vi "30XX.VI"() -> ()   [LabVIEW 2015]
uses:
  board.vis/Globals.vi
  <vilib>/Analysis/NI_AALBase.lvlib
panel:
  in  "send all":bool
  in  "Offset ADC 8":u16=49000
  in  "Offset ADC 3":u16=49000
  in  "Offset ADC 7":u16=49000
  in  "Offset ADC 2":u16=49000
  in  "Offset ADC 6":u16=49000
  in  "Offset ADC 1":u16=49000
  in  "Offset ADC 5":u16=49000
  in  "Offset ADC 4":u16=49000
  in  "custom pattern: 14bits (hex)":fxp<+,14,14>=100.0 format="%x"
  out "data adr  0x25":u16 format="%x"
  out "data adr  0x26":u16 format="%x"
  out "custom pattern: 14bits (dec)":fxp<+,14,14>
  in  "ADC mode":enum32{"1", "2", "3"}(radio)=enum."3"
  out "Signalverlaufgraph Cam 2":u16[](graph)=[28, 28, 29, 29, 30, 30, 31, 31, 32, 32, 33, 33, 34, 34, 35, 35, 36, 36, 37, 37, 38, 38, 39, 39, 40, 40, 41, 41, 42, 42, 43, 43, 44, 44, 45, 45, 46, 46, 47, 47, 48, 48, 49, 49, 50, 50, 51, 51, 52, 52, 53, 53, 54, 54, 55, 55, 56, 56, 57, 57, 58, 58, 59, 59, 60, 60, 61, 61, 62, 62, 63, 63, 64, 64, 65, 65, 66, 66, 67, 67, 68, 68, 69, 69, 70, 70, 71, 71, 72, 72, 73, 73, 74, 74, 75, 75, 76, 76, 77, 77, 78, 78, 79, 79, 80, 80, 81, 81, 82, 82, 83, 83, 84, 84, 85, 85, 86, 86, 87, 87, 88, 88, 89, 89, 90, 90, 91, 91, 92, 92, 93, 93, 94, 94, 95, 95, 96, 96, 97, 97, 98, 98, 99, 99, 100, 100, 101, 101, 102, 102, 103, 103, 104, 104, 105, 105, 106, 106, 107, 107, 108, 108, 109, 109, 110, 110, 111, 111, 112, 112, 113, 113, 114, 114, 115, 115, 116, 116, 117, 117, 118, 118, 119, 119, 120, 120, 121, 121, 122, 122, 123, 123, 124, 124, 125, 125, 126, 126, 127, 127, 128, 128, 129, 129, 130, 130, 131, 131, 132, 132, 133, 133, 134, 134, 135, 135, 136, 136, 137, 137, 138, 138, 139, 139, 140, 140, 141, 141, 142, 142, 143, 143, 144, 144, 145, 145, 146, 146, 147, 147, 148, 148, 149, 149, 150, 150, 151, 151, 152, 152, 153, 153, 154, 154, 155, 155, 156, 156, 157, 157, 158, 158, 159, 159, 160, 160, 161, 161, 162, 162, 163, 163, 164, 164, 165, 165, 166, 166, 167, 167, 168, 168, 169, 169, 170, 170, 171, 171, 172, 172, 173, 173, 174, 174, 175, 175, 176, 176, 177, 177, 178, 178, 179, 179, 180, 180, 181, 181, 182, 182, 183, 183, 184, 184, 185, 185, 186, 186, 187, 187, 188, 188, 189, 189, 190, 190, 191, 191, 192, 192, 193, 193, 194, 194, 195, 195, 196, 196, 197, 197, 198, 198, 199, 199, 200, 200, 201, 201, 202, 202, 203, 203, 204, 204, 205, 205, 206, 206, 207, 207, 208, 208, 209, 209, 210, 210, 211, 211, 212, 212, 213, 213, 214, 214, 215, 215, 216, 216, 217, 217, 218, 218, 219, 219, 220, 220, 221, 221, 222, 222, 223, 223, 224, 224, 225, 225, 226, 226, 227, 227, 228, 228, 229, 229, 230, 230, 231, 231, 232, 232, 233, 233, 234, 234, 235, 235, 236, 236, 237, 237, 238, 238, 239, 239, 240, 240, 241, 241, 242, 242, 243, 243, 244, 244, 245, 245, 246, 246, 247, 247, 248, 248, 249, 249, 250, 250, 251, 251, 252, 252, 253, 253, 254, 254, 255, 255, 256, 256, 257, 257, 258, 258, 259, 259, 260, 260, 261, 261, 262, 262, 263, 263, 264, 264, 265, 265, 266, 266, 267, 267, 268, 268, 269, 269, 270, 270, 271, 271, 272, 272, 273, 273, 274, 274, 275, 275, 276, 276, 277, 277, 278, 278, 279, 279, 280, 280, 281, 281, 282, 282, 283, 283, 284, 284, 285, 285, 286, 286, 287, 287, 288, 288, 289, 289, 290, 290, 291, 291, 292, 292, 293, 293, 294, 294, 295, 295, 296, 296, 297, 297, 298, 298, 299, 299, 300, 300, 301, 301, 302, 302, 303, 303, 304, 304, 305, 305, 306, 306, 307, 307, 308, 308, 309, 309, 310, 310, 311, 311, 312, 312, 313, 313, 314, 314, 315, 315, 316, 316, 317, 317, 318, 318, 319, 319, 320, 320, 321, 321, 322, 322, 323, 323, 324, 324, 325, 325, 326, 326, 327, 327, 328, 328, 329, 329, 330, 330, 331, 331, 332, 332, 333, 333, 334, 334, 335, 335, 336, 336, 337, 337, 338, 338, 339, 339, 340, 340, 341, 341, 342, 342, 343, 343, 344, 344, 345, 345, 346, 346, 347, 347, 348, 348, 349, 349, 350, 350, 351, 351, 352, 352, 353, 353, 354, 354, 355, 355, 356, 356, 357, 357, 358, 358, 359, 359, 360, 360, 361, 361, 362, 362, 363, 363, 364, 364, 365, 365, 366, 366, 367, 367, 368, 368, 369, 369, 370, 370, 371, 371, 372, 372, 373, 373, 374, 374, 375, 375, 376, 376, 377, 377, 378, 378, 379, 379, 380, 380, 381, 381, 382, 382, 383, 383, 384, 384, 385, 385, 386, 386, 387, 387, 388, 388, 389, 389, 390, 390, 391, 391, 392, 392, 393, 393, 394, 394, 395, 395, 396, 396, 397, 397, 398, 398, 399, 399, 400, 400, 401, 401, 402, 402, 403, 403, 404, 404, 405, 405, 406, 406, 407, 407, 408, 408, 409, 409, 410, 410, 411, 411, 412, 412, 413, 413, 414, 414, 415, 415, 416, 416, 417, 417, 418, 418, 419, 419, 420, 420, 421, 421, 422, 422, 423, 423, 424, 424, 425, 425, 426, 426, 427, 427, 428, 428, 429, 429, 430, 430, 431, 431, 432, 432, 433, 433, 434, 434, 435, 435, 436, 436, 437, 437, 438, 438, 439, 439, 440, 440, 441, 441, 442, 442, 443, 443, 444, 444, 445, 445, 446, 446, 447, 447, 448, 448, 449, 449, 450, 450, 451, 451, 452, 452, 453, 453, 454, 454, 455, 455, 456, 456, 457, 457, 458, 458, 459, 459, 460, 460, 461, 461, 462, 462, 463, 463, 464, 464, 465, 465, 466, 466, 467, 467, 468, 468, 469, 469, 470, 470, 471, 471, 472, 472, 473, 473, 474, 474, 475, 475, 476, 476, 477, 477, 478, 478, 479, 479, 480, 480, 481, 481, 482, 482, 483, 483, 484, 484, 485, 485, 486, 486, 487, 487, 488, 488, 489, 489, 490, 490, 491, 491, 492, 492, 493, 493, 494, 494, 495, 495, 496, 496, 497, 497, 498, 498, 499, 499, 500, 500, 501, 501, 502, 502, 503, 503, 504, 504, 505, 505, 506, 506, 507, 507, 508, 508, 509, 509, 510, 510, 511, 511, 512, 512, 513, 513, 514, 514, 515, 515, 516, 516, 517, 517, 518, 518, 519, 519, 520, 520, 521, 521, 522, 522, 523, 523, 524, 524, 525, 525, 526, 526, 527, 527, 528, 528, 529, 529, 530, 530, 531, 531, 532, 532, 533, 533, 534, 534, 535, 535, 536, 536, 537, 537, 538, 538, 539, 539, 540, 540, 541, 541, 542, 542, 543, 543, 544, 544, 544, 544, 544, 544, 544, 544, 544, 544, 544, 544, 544, 544, 544, 544, 544, 544, 544, 544, 544, 544, 544, 544, 544, 544, 544, 544, 544, 544, 544, 544, 544, 544, 544, 544, 544, 544, 544, 544, 544, 544, 544, 544, 544, 544, 544, 544, 544, 544, 544, 544, 544, 544, 544, 544]
  in  "extTrig":bool
  in  "ext. trig. slope":enum32{"1", "2", "3"}(radio)
  out "tRMS":dbl format="%0#.1f"
  out "mean":dbl=100.0 format="%#_4f"
  in  "rms_pixel":u16=100
  in  "is FFT":bool=TRUE
  in  "IR gain":bool
  in  "continuous":bool
  out "curr.block":u8=2
  out "Measure ON":bool
  in  "Board select\n1: board 1\n2: board 2\n3: both boards":u8=3
  in  "no.of blocks (nob)\npress enter":u32=4
  in  "block":u32(slide)=2 max=10 scale=0.9..4.0
  out "Signalverlaufgraph Board 2":u16[](graph)=[0, 0, 543, 543, 0, 1, 0, 0, 2, 2, 3, 3, 4, 4, 5, 5, 6, 6, 7, 7, 8, 8, 9, 9, 10, 10, 11, 11, 12, 12, 13, 13, 14, 14, 15, 15, 16, 16, 17, 17, 18, 18, 19, 19, 20, 20, 21, 21, 22, 22, 23, 23, 24, 24, 25, 25, 26, 26, 27, 27, 28, 28, 29, 29, 30, 30, 31, 31, 32, 32, 33, 33, 34, 34, 35, 35, 36, 36, 37, 37, 38, 38, 39, 39, 40, 40, 41, 41, 42, 42, 43, 43, 44, 44, 45, 45, 46, 46, 47, 47, 48, 48, 49, 49, 50, 50, 51, 51, 52, 52, 53, 53, 54, 54, 55, 55, 56, 56, 57, 57, 58, 58, 59, 59, 60, 60, 61, 61, 62, 62, 63, 63, 64, 64, 65, 65, 66, 66, 67, 67, 68, 68, 69, 69, 70, 70, 71, 71, 72, 72, 73, 73, 74, 74, 75, 75, 76, 76, 77, 77, 78, 78, 79, 79, 80, 80, 81, 81, 82, 82, 83, 83, 84, 84, 85, 85, 86, 86, 87, 87, 88, 88, 89, 89, 90, 90, 91, 91, 92, 92, 93, 93, 94, 94, 95, 95, 96, 96, 97, 97, 98, 98, 99, 99, 100, 100, 101, 101, 102, 102, 103, 103, 104, 104, 105, 105, 106, 106, 107, 107, 108, 108, 109, 109, 110, 110, 111, 111, 112, 112, 113, 113, 114, 114, 115, 115, 116, 116, 117, 117, 118, 118, 119, 119, 120, 120, 121, 121, 122, 122, 123, 123, 124, 124, 125, 125, 126, 126, 127, 127, 128, 128, 129, 129, 130, 130, 131, 131, 132, 132, 133, 133, 134, 134, 135, 135, 136, 136, 137, 137, 138, 138, 139, 139, 140, 140, 141, 141, 142, 142, 143, 143, 144, 144, 145, 145, 146, 146, 147, 147, 148, 148, 149, 149, 150, 150, 151, 151, 152, 152, 153, 153, 154, 154, 155, 155, 156, 156, 157, 157, 158, 158, 159, 159, 160, 160, 161, 161, 162, 162, 163, 163, 164, 164, 165, 165, 166, 166, 167, 167, 168, 168, 169, 169, 170, 170, 171, 171, 172, 172, 173, 173, 174, 174, 175, 175, 176, 176, 177, 177, 178, 178, 179, 179, 180, 180, 181, 181, 182, 182, 183, 183, 184, 184, 185, 185, 186, 186, 187, 187, 188, 188, 189, 189, 190, 190, 191, 191, 192, 192, 193, 193, 194, 194, 195, 195, 196, 196, 197, 197, 198, 198, 199, 199, 200, 200, 201, 201, 202, 202, 203, 203, 204, 204, 205, 205, 206, 206, 207, 207, 208, 208, 209, 209, 210, 210, 211, 211, 212, 212, 213, 213, 214, 214, 215, 215, 216, 216, 217, 217, 218, 218, 219, 219, 220, 220, 221, 221, 222, 222, 223, 223, 224, 224, 225, 225, 226, 226, 227, 227, 228, 228, 229, 229, 230, 230, 231, 231, 232, 232, 233, 233, 234, 234, 235, 235, 236, 236, 237, 237, 238, 238, 239, 239, 240, 240, 241, 241, 242, 242, 243, 243, 244, 244, 245, 245, 246, 246, 247, 247, 248, 248, 249, 249, 250, 250, 251, 251, 252, 252, 253, 253, 254, 254, 255, 255, 256, 256, 257, 257, 258, 258, 259, 259, 260, 260, 261, 261, 262, 262, 263, 263, 264, 264, 265, 265, 266, 266, 267, 267, 268, 268, 269, 269, 270, 270, 271, 271, 272, 272, 273, 273, 274, 274, 275, 275, 276, 276, 277, 277, 278, 278, 279, 279, 280, 280, 281, 281, 282, 282, 283, 283, 284, 284, 285, 285, 286, 286, 287, 287, 288, 288, 289, 289, 290, 290, 291, 291, 292, 292, 293, 293, 294, 294, 295, 295, 296, 296, 297, 297, 298, 298, 299, 299, 300, 300, 301, 301, 302, 302, 303, 303, 304, 304, 305, 305, 306, 306, 307, 307, 308, 308, 309, 309, 310, 310, 311, 311, 312, 312, 313, 313, 314, 314, 315, 315, 316, 316, 317, 317, 318, 318, 319, 319, 320, 320, 321, 321, 322, 322, 323, 323, 324, 324, 325, 325, 326, 326, 327, 327, 328, 328, 329, 329, 330, 330, 331, 331, 332, 332, 333, 333, 334, 334, 335, 335, 336, 336, 337, 337, 338, 338, 339, 339, 340, 340, 341, 341, 342, 342, 343, 343, 344, 344, 345, 345, 346, 346, 347, 347, 348, 348, 349, 349, 350, 350, 351, 351, 352, 352, 353, 353, 354, 354, 355, 355, 356, 356, 357, 357, 358, 358, 359, 359, 360, 360, 361, 361, 362, 362, 363, 363, 364, 364, 365, 365, 366, 366, 367, 367, 368, 368, 369, 369, 370, 370, 371, 371, 372, 372, 373, 373, 374, 374, 375, 375, 376, 376, 377, 377, 378, 378, 379, 379, 380, 380, 381, 381, 382, 382, 383, 383, 384, 384, 385, 385, 386, 386, 387, 387, 388, 388, 389, 389, 390, 390, 391, 391, 392, 392, 393, 393, 394, 394, 395, 395, 396, 396, 397, 397, 398, 398, 399, 399, 400, 400, 401, 401, 402, 402, 403, 403, 404, 404, 405, 405, 406, 406, 407, 407, 408, 408, 409, 409, 410, 410, 411, 411, 412, 412, 413, 413, 414, 414, 415, 415, 416, 416, 417, 417, 418, 418, 419, 419, 420, 420, 421, 421, 422, 422, 423, 423, 424, 424, 425, 425, 426, 426, 427, 427, 428, 428, 429, 429, 430, 430, 431, 431, 432, 432, 433, 433, 434, 434, 435, 435, 436, 436, 437, 437, 438, 438, 439, 439, 440, 440, 441, 441, 442, 442, 443, 443, 444, 444, 445, 445, 446, 446, 447, 447, 448, 448, 449, 449, 450, 450, 451, 451, 452, 452, 453, 453, 454, 454, 455, 455, 456, 456, 457, 457, 458, 458, 459, 459, 460, 460, 461, 461, 462, 462, 463, 463, 464, 464, 465, 465, 466, 466, 467, 467, 468, 468, 469, 469, 470, 470, 471, 471, 472, 472, 473, 473, 474, 474, 475, 475, 476, 476, 477, 477, 478, 478, 479, 479, 480, 480, 481, 481, 482, 482, 483, 483, 484, 484, 485, 485, 486, 486, 487, 487, 488, 488, 489, 489, 490, 490, 491, 491, 492, 492, 493, 493, 494, 494, 495, 495, 496, 496, 497, 497, 498, 498, 499, 499, 500, 500, 501, 501, 502, 502, 503, 503, 504, 504, 505, 505, 506, 506, 507, 507, 508, 508, 509, 509, 510, 510, 511, 511, 512, 512, 513, 513, 514, 514, 515, 515, 516, 516, 517, 517, 518, 518, 519, 519, 520, 520, 521, 521, 522, 522, 523, 523, 524, 524, 525, 525, 526, 526, 527, 527, 528, 528, 529, 529, 530, 530, 531, 531, 532, 532, 533, 533, 534, 534, 535, 535, 536, 536, 537, 537, 538, 538, 539, 539, 540, 540, 541, 541]
  out "Signalverlaufgraph":u16[](graph)=[544, 544, 545, 545, 49152, 2, 0, 762, 2, 2, 3, 3, 4, 4, 5, 5, 6, 6, 7, 7, 8, 8, 9, 9, 10, 10, 11, 11, 12, 12, 13, 13, 14, 14, 15, 15, 16, 16, 17, 17, 18, 18, 19, 19, 20, 20, 21, 21, 22, 22, 23, 23, 24, 24, 25, 25, 26, 26, 27, 27, 28, 28, 29, 29, 30, 30, 31, 31, 32, 32, 33, 33, 34, 34, 35, 35, 36, 36, 37, 37, 38, 38, 39, 39, 40, 40, 41, 41, 42, 42, 43, 43, 44, 44, 45, 45, 46, 46, 47, 47, 48, 48, 49, 49, 50, 50, 51, 51, 52, 52, 53, 53, 54, 54, 55, 55, 56, 56, 57, 57, 58, 58, 59, 59, 60, 60, 61, 61, 62, 62, 63, 63, 64, 64, 65, 65, 66, 66, 67, 67, 68, 68, 69, 69, 70, 70, 71, 71, 72, 72, 73, 73, 74, 74, 75, 75, 76, 76, 77, 77, 78, 78, 79, 79, 80, 80, 81, 81, 82, 82, 83, 83, 84, 84, 85, 85, 86, 86, 87, 87, 88, 88, 89, 89, 90, 90, 91, 91, 92, 92, 93, 93, 94, 94, 95, 95, 96, 96, 97, 97, 98, 98, 99, 99, 100, 100, 101, 101, 102, 102, 103, 103, 104, 104, 105, 105, 106, 106, 107, 107, 108, 108, 109, 109, 110, 110, 111, 111, 112, 112, 113, 113, 114, 114, 115, 115, 116, 116, 117, 117, 118, 118, 119, 119, 120, 120, 121, 121, 122, 122, 123, 123, 124, 124, 125, 125, 126, 126, 127, 127, 128, 128, 129, 129, 130, 130, 131, 131, 132, 132, 133, 133, 134, 134, 135, 135, 136, 136, 137, 137, 138, 138, 139, 139, 140, 140, 141, 141, 142, 142, 143, 143, 144, 144, 145, 145, 146, 146, 147, 147, 148, 148, 149, 149, 150, 150, 151, 151, 152, 152, 153, 153, 154, 154, 155, 155, 156, 156, 157, 157, 158, 158, 159, 159, 160, 160, 161, 161, 162, 162, 163, 163, 164, 164, 165, 165, 166, 166, 167, 167, 168, 168, 169, 169, 170, 170, 171, 171, 172, 172, 173, 173, 174, 174, 175, 175, 176, 176, 177, 177, 178, 178, 179, 179, 180, 180, 181, 181, 182, 182, 183, 183, 184, 184, 185, 185, 186, 186, 187, 187, 188, 188, 189, 189, 190, 190, 191, 191, 192, 192, 193, 193, 194, 194, 195, 195, 196, 196, 197, 197, 198, 198, 199, 199, 200, 200, 201, 201, 202, 202, 203, 203, 204, 204, 205, 205, 206, 206, 207, 207, 208, 208, 209, 209, 210, 210, 211, 211, 212, 212, 213, 213, 214, 214, 215, 215, 216, 216, 217, 217, 218, 218, 219, 219, 220, 220, 221, 221, 222, 222, 223, 223, 224, 224, 225, 225, 226, 226, 227, 227, 228, 228, 229, 229, 230, 230, 231, 231, 232, 232, 233, 233, 234, 234, 235, 235, 236, 236, 237, 237, 238, 238, 239, 239, 240, 240, 241, 241, 242, 242, 243, 243, 244, 244, 245, 245, 246, 246, 247, 247, 248, 248, 249, 249, 250, 250, 251, 251, 252, 252, 253, 253, 254, 254, 255, 255, 256, 256, 257, 257, 258, 258, 259, 259, 260, 260, 261, 261, 262, 262, 263, 263, 264, 264, 265, 265, 266, 266, 267, 267, 268, 268, 269, 269, 270, 270, 271, 271, 272, 272, 273, 273, 274, 274, 275, 275, 276, 276, 277, 277, 278, 278, 279, 279, 280, 280, 281, 281, 282, 282, 283, 283, 284, 284, 285, 285, 286, 286, 287, 287, 288, 288, 289, 289, 290, 290, 291, 291, 292, 292, 293, 293, 294, 294, 295, 295, 296, 296, 297, 297, 298, 298, 299, 299, 300, 300, 301, 301, 302, 302, 303, 303, 304, 304, 305, 305, 306, 306, 307, 307, 308, 308, 309, 309, 310, 310, 311, 311, 312, 312, 313, 313, 314, 314, 315, 315, 316, 316, 317, 317, 318, 318, 319, 319, 320, 320, 321, 321, 322, 322, 323, 323, 324, 324, 325, 325, 326, 326, 327, 327, 328, 328, 329, 329, 330, 330, 331, 331, 332, 332, 333, 333, 334, 334, 335, 335, 336, 336, 337, 337, 338, 338, 339, 339, 340, 340, 341, 341, 342, 342, 343, 343, 344, 344, 345, 345, 346, 346, 347, 347, 348, 348, 349, 349, 350, 350, 351, 351, 352, 352, 353, 353, 354, 354, 355, 355, 356, 356, 357, 357, 358, 358, 359, 359, 360, 360, 361, 361, 362, 362, 363, 363, 364, 364, 365, 365, 366, 366, 367, 367, 368, 368, 369, 369, 370, 370, 371, 371, 372, 372, 373, 373, 374, 374, 375, 375, 376, 376, 377, 377, 378, 378, 379, 379, 380, 380, 381, 381, 382, 382, 383, 383, 384, 384, 385, 385, 386, 386, 387, 387, 388, 388, 389, 389, 390, 390, 391, 391, 392, 392, 393, 393, 394, 394, 395, 395, 396, 396, 397, 397, 398, 398, 399, 399, 400, 400, 401, 401, 402, 402, 403, 403, 404, 404, 405, 405, 406, 406, 407, 407, 408, 408, 409, 409, 410, 410, 411, 411, 412, 412, 413, 413, 414, 414, 415, 415, 416, 416, 417, 417, 418, 418, 419, 419, 420, 420, 421, 421, 422, 422, 423, 423, 424, 424, 425, 425, 426, 426, 427, 427, 428, 428, 429, 429, 430, 430, 431, 431, 432, 432, 433, 433, 434, 434, 435, 435, 436, 436, 437, 437, 438, 438, 439, 439, 440, 440, 441, 441, 442, 442, 443, 443, 444, 444, 445, 445, 446, 446, 447, 447, 448, 448, 449, 449, 450, 450, 451, 451, 452, 452, 453, 453, 454, 454, 455, 455, 456, 456, 457, 457, 458, 458, 459, 459, 460, 460, 461, 461, 462, 462, 463, 463, 464, 464, 465, 465, 466, 466, 467, 467, 468, 468, 469, 469, 470, 470, 471, 471, 472, 472, 473, 473, 474, 474, 475, 475, 476, 476, 477, 477, 478, 478, 479, 479, 480, 480, 481, 481, 482, 482, 483, 483, 484, 484, 485, 485, 486, 486, 487, 487, 488, 488, 489, 489, 490, 490, 491, 491, 492, 492, 493, 493, 494, 494, 495, 495, 496, 496, 497, 497, 498, 498, 499, 499, 500, 500, 501, 501, 502, 502, 503, 503, 504, 504, 505, 505, 506, 506, 507, 507, 508, 508, 509, 509, 510, 510, 511, 511, 512, 512, 513, 513, 514, 514, 515, 515, 516, 516, 517, 517, 518, 518, 519, 519, 520, 520, 521, 521, 522, 522, 523, 523, 524, 524, 525, 525, 526, 526, 527, 527, 528, 528, 529, 529, 530, 530, 531, 531, 532, 532, 533, 533, 534, 534, 535, 535, 536, 536, 537, 537, 538, 538, 539, 539, 540, 540, 541, 541]
  out "boards recognised":u8=1
  in  "alloc mem":bool
  out "FREE \nRAM MB":dbl=15821.3046875
  out "BUILT-IN\nRAM MB":dbl=18096.171875
  out "SEC":dbl=0.44
  out "MB RAM":dbl=18.26171875
  in  "DAT in 10ns":u32
  in  "stop all":bool
  in  "start":bool
  in  "sample":u32(slide)=382 max=3000 scale=0.9..1100.0
  in  "no.of samples (nos)":u32=1100
  in  "exposuretime[ms]":dbl=0.1 format="%.3f"
  # "press Esc to stop measurement"
  # "exit here"
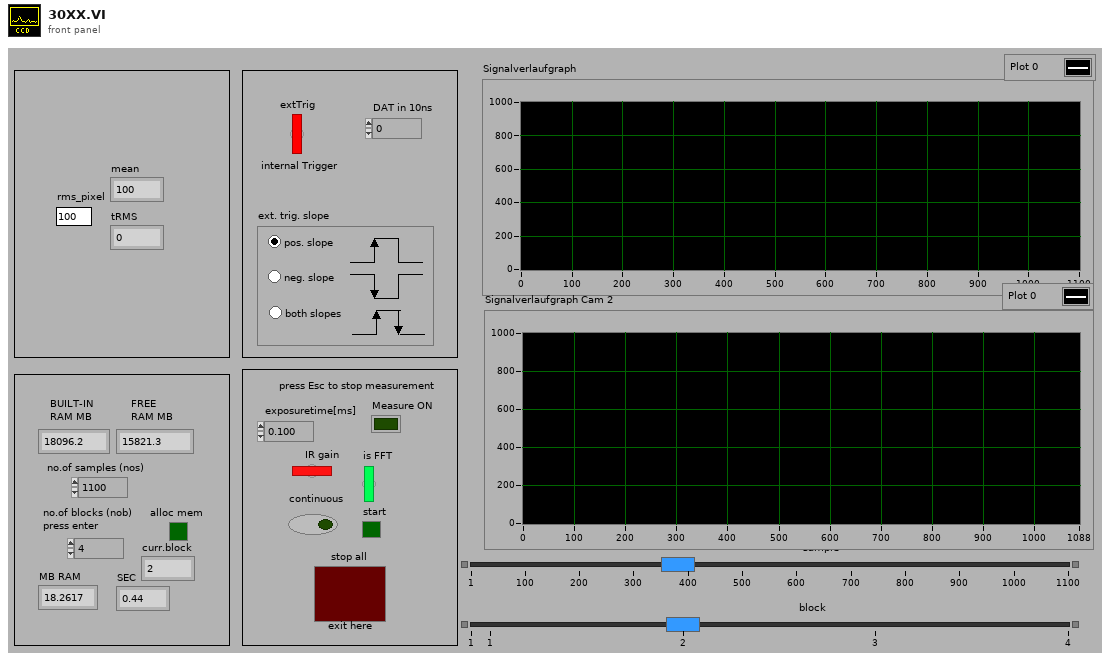
[diagram p1: front panel]
types:
  T1 = enum8{"Enabled", "Disabled", "Disabled and Grayed Out"}
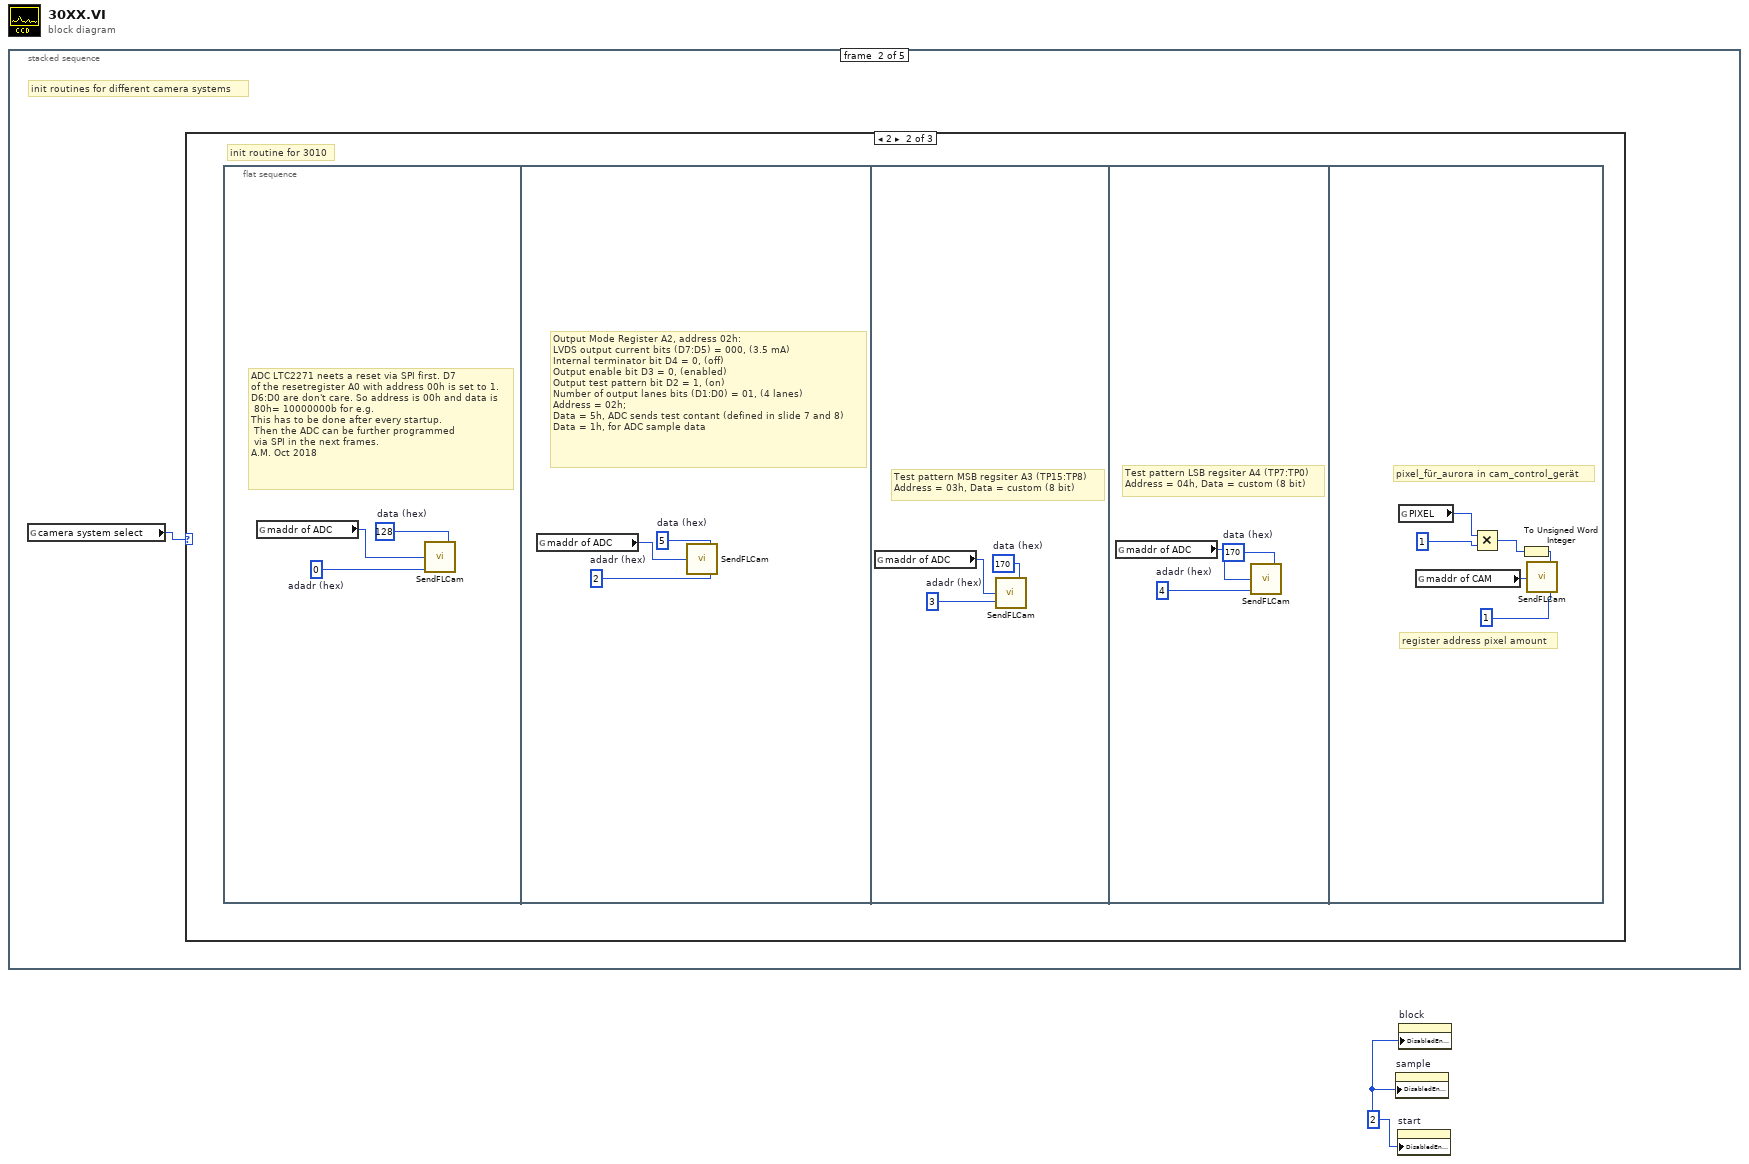
[diagram p0: block diagram]
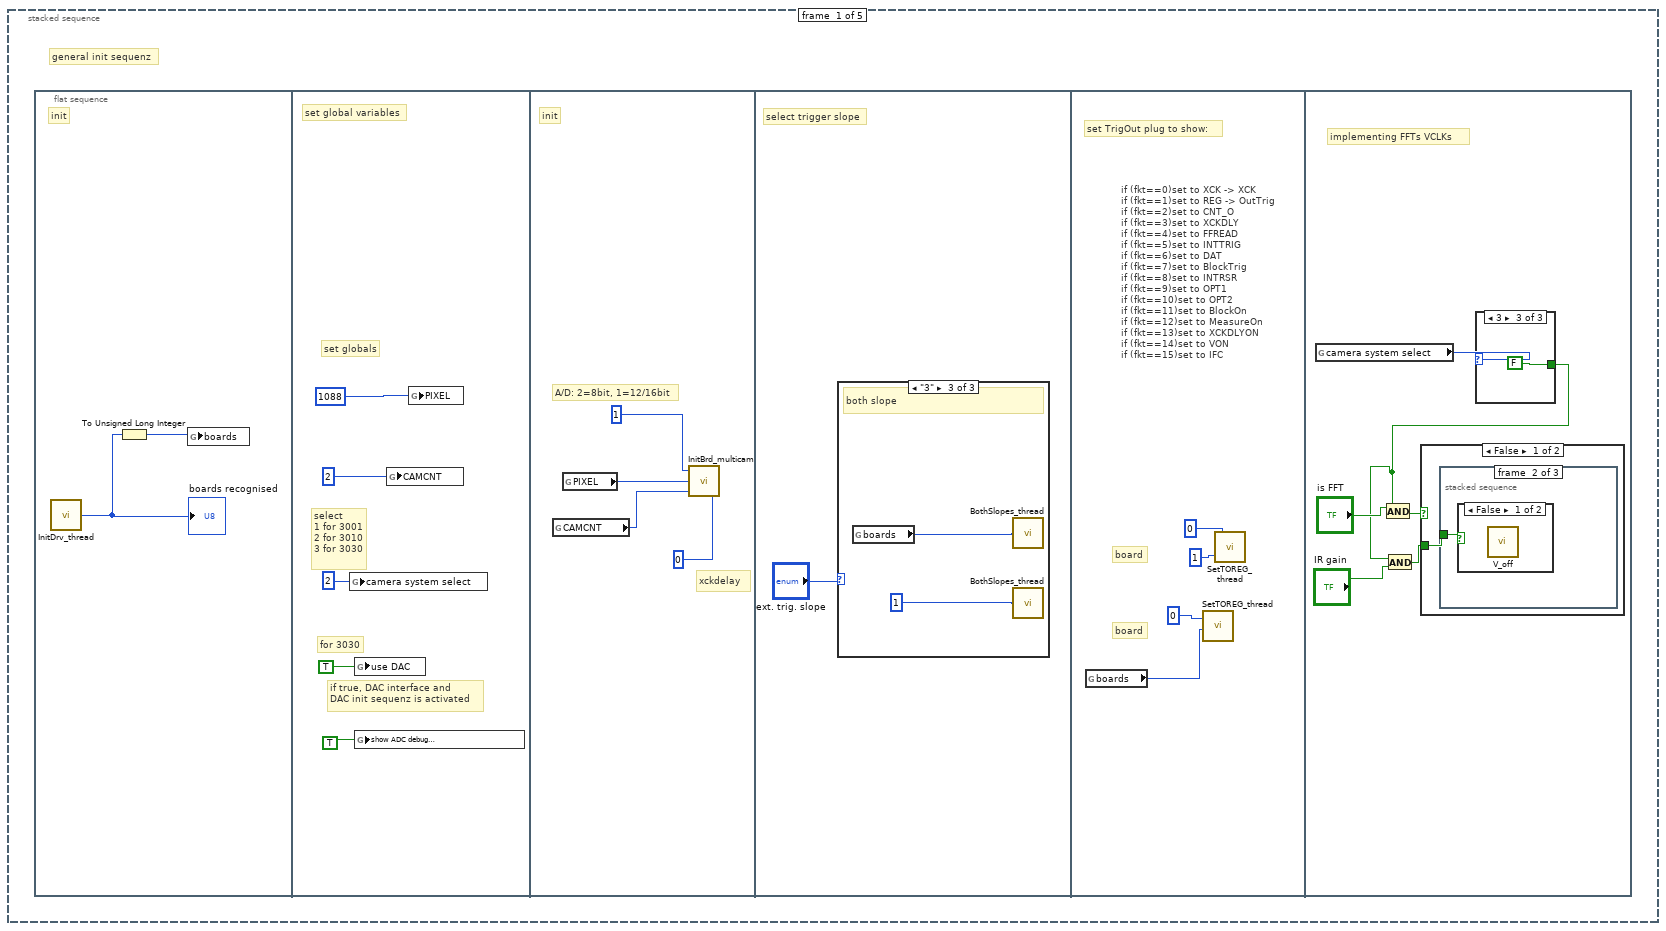
[diagram p2: hidden frame]
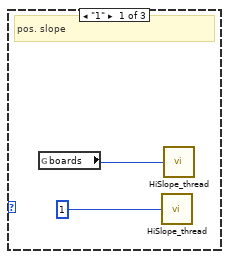
[diagram p3: hidden frame]
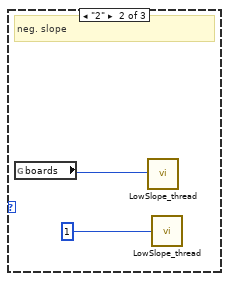
[diagram p4: hidden frame]
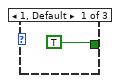
[diagram p5: hidden frame]
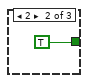
[diagram p6: hidden frame]
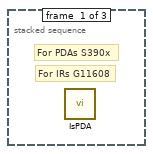
[diagram p7: hidden frame]
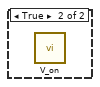
[diagram p8: hidden frame]
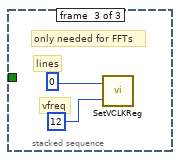
[diagram p9: hidden frame]
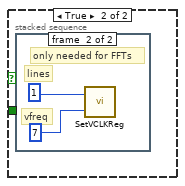
[diagram p10: hidden frame]
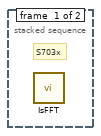
[diagram p11: hidden frame]
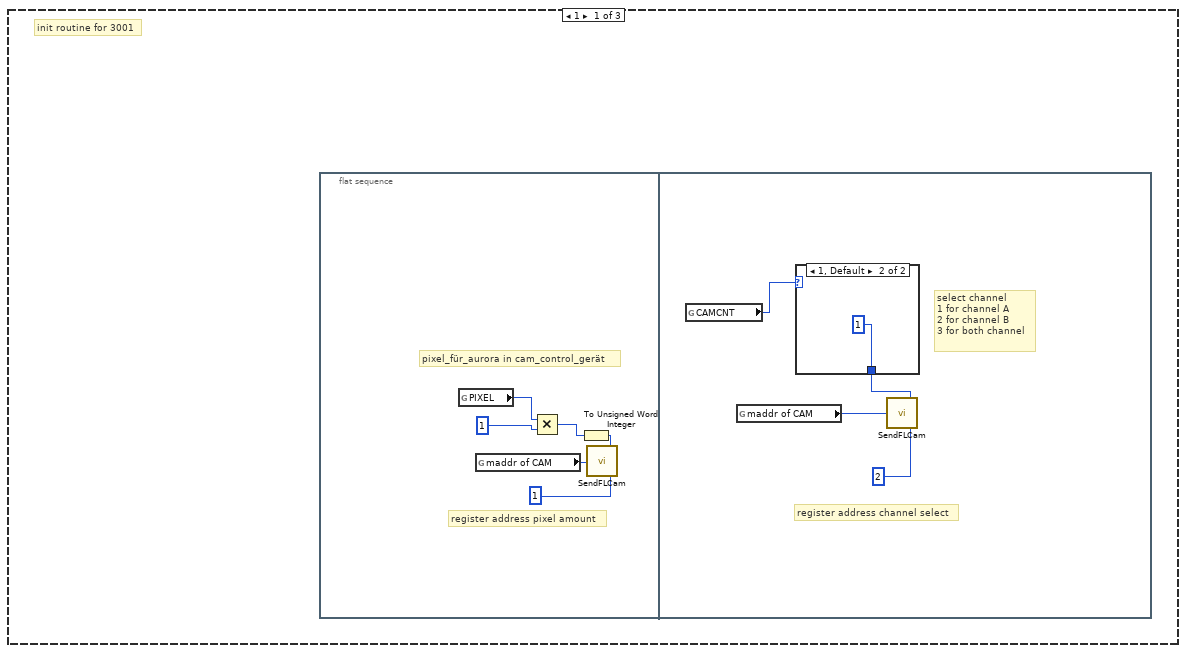
[diagram p12: hidden frame]
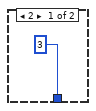
[diagram p13: hidden frame]
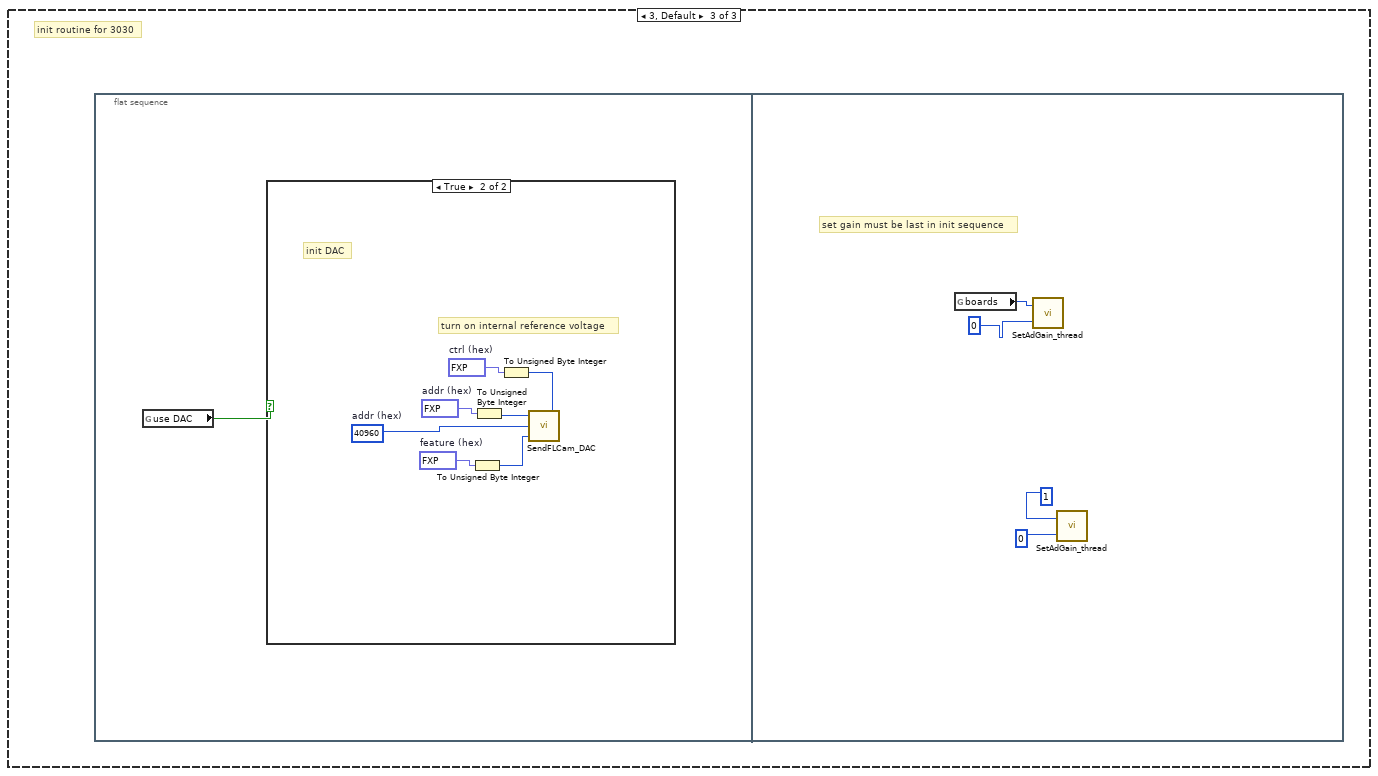
[diagram p14: hidden frame]
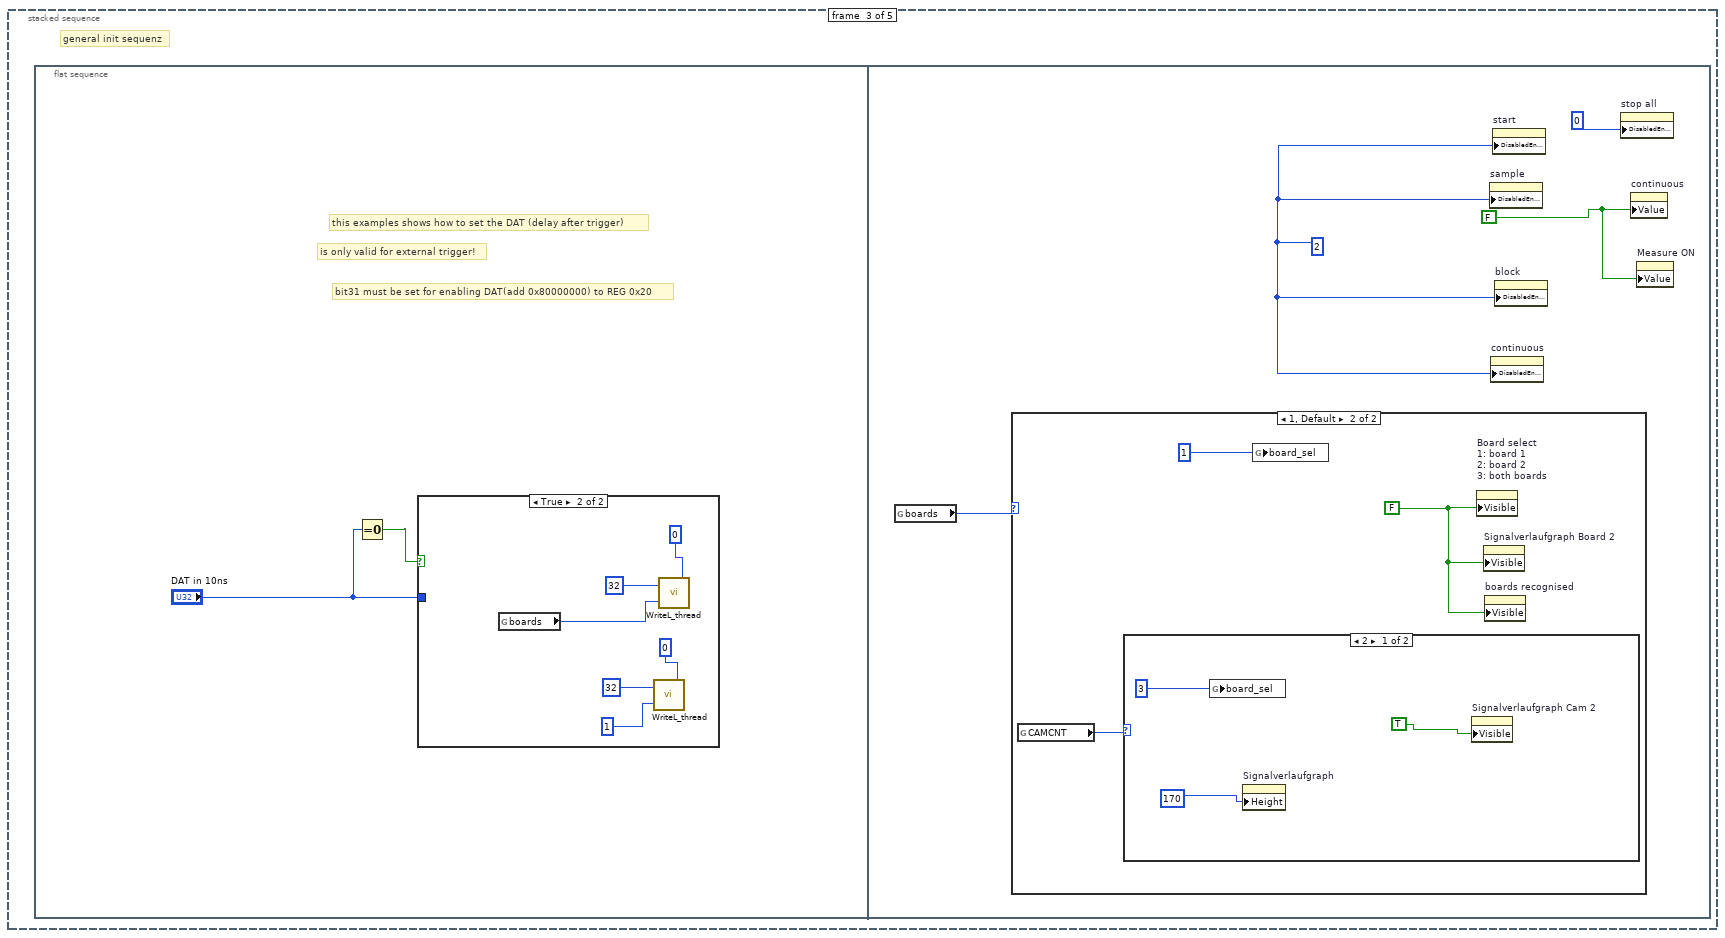
[diagram p16: hidden frame]
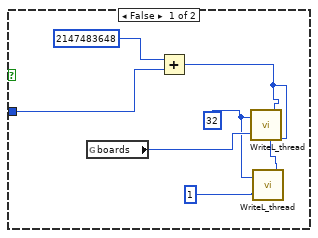
[diagram p17: hidden frame]
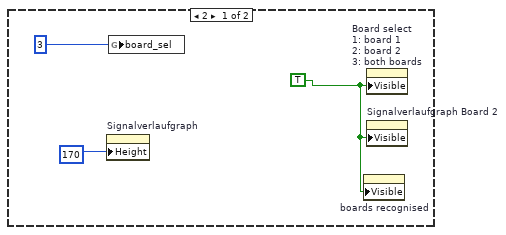
[diagram p18: hidden frame]
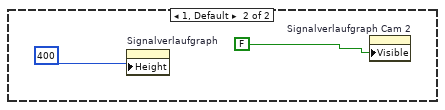
[diagram p19: hidden frame]
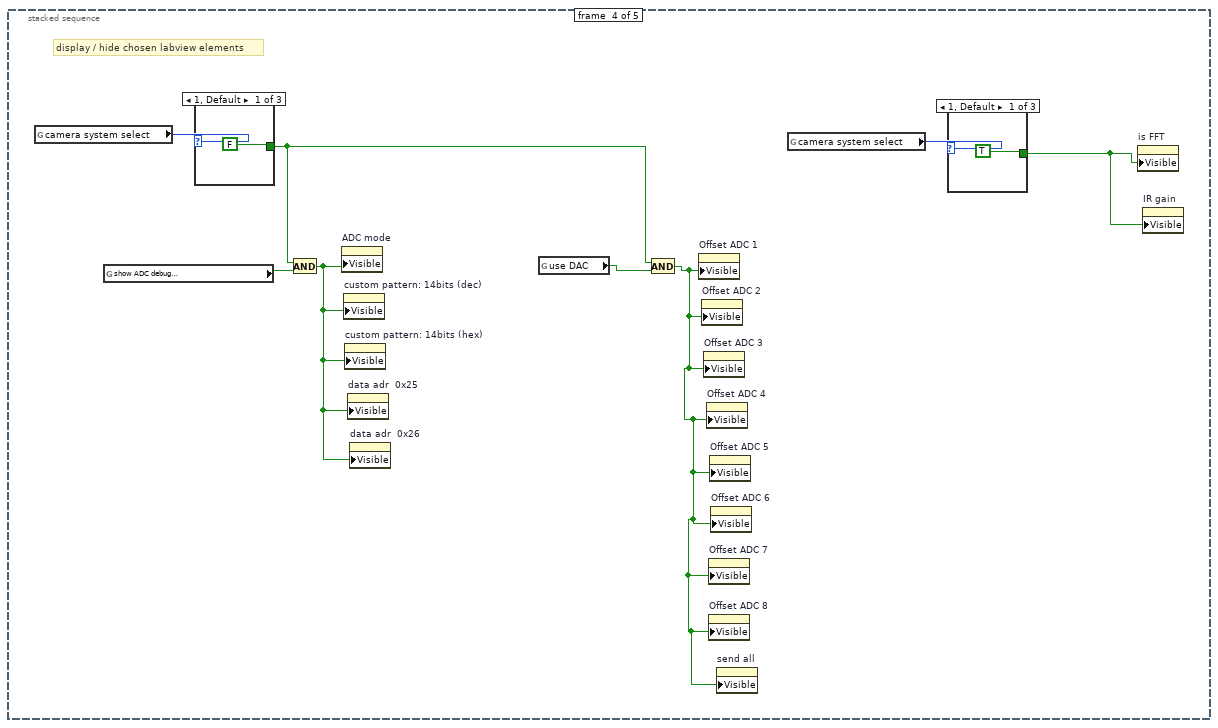
[diagram p20: hidden frame]
diagram:
  w1 = 2
  n1 = stacked-sequence {
    frame #0 {
      # "general init sequenz"
      n2 = flat-sequence {
        frame #0 {
          # "init"
          n3 = call "InitDrv_thread.vi"() -> ("Boards"=w2:u8)  [unwired: 1 in]
          "boards recognised" <- w2
          n4 = To Unsigned Long Integer(number=w2) -> (unsigned 32bit integer=w3:u32)
          n5 = global write "Globals.vi" "boards"(w3) -> ()
        }
        frame #1 {
          # "if true, DAC interface and \nDAC init sequenz is activated"
          # "for 3030"
          # "set global variables"
          # "select \n1 for 3001\n2 for 3010\n3 for 3030"
          # "set globals"
          n6 = global write "Globals.vi" "camera system select"(u8 2) -> ()
          n7 = global write "Globals.vi" "use DAC"(TRUE) -> ()
          n8 = global write "Globals.vi" "show ADC debug \ninterface"(TRUE) -> ()
          n9 = global write "Globals.vi" "CAMCNT"(u32 2) -> ()
          n10 = global write "Globals.vi" "PIXEL"(u32 1088) -> ()
        }
        frame #2 {
          # "init"
          # "xckdelay"
          # "A/D: 2=8bit, 1=12/16bit"
          n11 = global read "Globals.vi" "CAMCNT"() -> (w9:u32)
          n12 = global read "Globals.vi" "PIXEL"() -> (w12:u32)
          n13 = call "InitBrd_multicam.vi"("xckdly"=u32 0, "camcnt"=w9, "pixel"=w12, "flag816"=u32 1) -> ()  [unwired: 2 in]
        }
        frame #3 {
          # "select trigger slope"
          n14 = case shown="\"3\"" "ext. trig. slope" {
            frame "1" {
              # "pos. slope"
              n15 = global read "Globals.vi" "boards"() -> (w14:u32)
              n16 = call "HiSlope_thread.vi"("board"=u32 1) -> ()  [unwired: 1 in]
              n17 = call "HiSlope_thread.vi"("board"=w14) -> ()  [unwired: 1 in]
            }
            frame "2" {
              # "neg. slope"
              n18 = global read "Globals.vi" "boards"() -> (w17:u32)
              n19 = call "LowSlope_thread.vi"("board"=w17) -> ()  [unwired: 1 in]
              n20 = call "LowSlope_thread.vi"("board"=u32 1) -> ()  [unwired: 1 in]
            }
            frame "3" {
              # "both slope"
              n21 = global read "Globals.vi" "boards"() -> (w18:u32)
              n22 = call "BothSlopes_thread.vi"("board"=w18) -> ()  [unwired: 1 in]
              n23 = call "BothSlopes_thread.vi"("board"=u32 1) -> ()  [unwired: 1 in]
            }
          }
        }
        frame #4 {
          # "if (fkt==0)set to XCK -> XCK\nif (fkt==1)set to REG -> OutTrig\nif (fkt==2)set to CNT_O\nif (fkt==3)set to XCKDLY\nif (fkt==4)set to FFREAD\nif (fkt==5)set to INTTRIG\nif (fkt==6)set to DAT\nif (fkt==7)set to BlockTrig\nif (fkt==8)set to INTRSR\nif (fkt==9)set to OPT1\nif (fkt==10)set to OPT2\nif (fkt==11)set to BlockOn\nif (fkt==12)set to MeasureOn\nif (fkt==13)set to XCKDLYON \nif (fkt==14)set to VON         \nif (fkt==15)set to IFC"
          # "board"
          # "board"
          # "set TrigOut plug to show:"
          n24 = global read "Globals.vi" "boards"() -> (w23:u32)
          n25 = call "SetTOREG_thread.vi"("board"=w23, "fkt"=u8 0) -> ()  [unwired: 1 in]
          n26 = call "SetTOREG_thread.vi"("board"=u32 1, "fkt"=u8 0) -> ()  [unwired: 1 in]
        }
        frame #5 {
          # "implementing FFTs VCLKs"
          n27 = global read "Globals.vi" "camera system select"() -> (w29:u8)
          n28 = case shown="3" w29 {
            tunnel: [TRUE TRUE FALSE] -> w24
            frame 1, Default {
            }
            frame 2 {
            }
            frame 3 {
            }
          }
          n29 = And(x="is FFT", y=w24) -> (x .and. y?=w28:bool)
          n30 = And(x=w24, y="IR gain") -> (x .and. y?=w26:bool)
          n31 = case shown="False" w28 {
            tunnel: w26 -> [w33 _]
            frame False {
              n32 = stacked-sequence {
                tunnel: w33 -> [_ w34 _]
                frame #0 {
                  # "For IRs G11608"
                  # "For PDAs S390x"
                  n33 = call "IsPDA.vi"() -> ()  [unwired: 1 in]
                }
                frame #1 {
                  n34 = case shown="False" w34 {
                    frame False {
                      n35 = call "V_off.vi"() -> ()  [unwired: 1 in]
                    }
                    frame True {
                      n36 = call "V_on.vi"() -> ()  [unwired: 1 in]
                    }
                  }
                }
                frame #2 {
                  # "only needed for FFTs"
                  # "vfreq"
                  # "lines"
                  n37 = call "SetVCLKReg.vi"("vfreq"=u8 12, "lines"=u32 0) -> ()  [unwired: 1 in]
                }
              }
            }
            frame True {
              n38 = stacked-sequence {
                frame #0 {
                  # "S703x"
                  n39 = call "IsFFT.vi"() -> ()  [unwired: 1 in]
                }
                frame #1 {
                  # "only needed for FFTs"
                  # "vfreq"
                  # "lines"
                  n40 = call "SetVCLKReg.vi"("vfreq"=u8 7, "lines"=u32 1) -> ()  [unwired: 1 in]
                }
              }
            }
          }
        }
      }
    }
    frame #1 {
      # "init routines for different camera systems"
      n41 = global read "Globals.vi" "camera system select"() -> (w39:u8)
      n42 = case shown="2" w39 {
        frame 1 {
          # "init routine for 3001"
          n43 = flat-sequence {
            frame #0 {
              # "register address pixel amount"
              # "pixel_für_aurora in cam_control_gerät"
              n44 = global read "Globals.vi" "PIXEL"() -> (w44:u32)
              n45 = global read "Globals.vi" "maddr of CAM"() -> (w41:u8)
              n46 = Multiply(x=w44, y=u32 1) -> (x*y=w43:u32)
              n47 = To Unsigned Word Integer(number=w43) -> (unsigned 16bit integer=w42:u16)
              n48 = call "SendFLCam.vi"("madr"=w41, "data"=w42, "adadr"=u8 1) -> ()
            }
            frame #1 {
              # "select channel\n1 for channel A\n2 for channel B\n3 for both channel"
              # "register address channel select"
              n49 = global read "Globals.vi" "CAMCNT"() -> (w47:u32)
              n50 = global read "Globals.vi" "maddr of CAM"() -> (w49:u8)
              n51 = case shown="1, Default" w47 {
                tunnel: [u16 3 u16 1] -> w46
                frame 2 {
                }
                frame 1, Default {
                }
              }
              n52 = call "SendFLCam.vi"("madr"=w49, "data"=w46, "adadr"=u8 2) -> ()
            }
          }
        }
        frame 2 {
          # "init routine for 3010"
          n53 = flat-sequence {
            frame #0 {
              w54 = u16 128  # data (hex)
              w53 = u8 0  # adadr (hex)
              # "ADC LTC2271 neets a reset via SPI first. D7\nof the resetregister A0 with address 00h is set to 1.\nD6:D0 are don't care. So address is 00h and data is\n 80h= 10000000b for e.g.  \nThis has to be done after every startup.\n Then the ADC can be further programmed\n via SPI in the next frames.\nA.M. Oct 2018"
              n54 = global read "Globals.vi" "maddr of ADC"() -> (w52:u8)
              n55 = call "SendFLCam.vi"("madr"=w52, "data"=w54, "adadr"=w53) -> ()
            }
            frame #1 {
              w56 = u16 5  # data (hex)
              w57 = u8 2  # adadr (hex)
              # "Output Mode Register A2, address 02h:\nLVDS output current bits (D7:D5) = 000, (3.5 mA)\nInternal terminator bit D4 = 0, (off)\nOutput enable bit D3 = 0, (enabled)\nOutput test pattern bit D2 = 1, (on)\nNumber of output lanes bits (D1:D0) = 01, (4 lanes)\nAddress = 02h;\nData = 5h, ADC sends test contant (defined in slide 7 and 8)\nData = 1h, for ADC sample data"
              n56 = global read "Globals.vi" "maddr of ADC"() -> (w55:u8)
              n57 = call "SendFLCam.vi"("madr"=w55, "data"=w56, "adadr"=w57) -> ()
            }
            frame #2 {
              w59 = u16 170  # data (hex)
              w60 = u8 3  # adadr (hex)
              # "Test pattern MSB regsiter A3 (TP15:TP8)\nAddress = 03h, Data = custom (8 bit)"
              n58 = global read "Globals.vi" "maddr of ADC"() -> (w58:u8)
              n59 = call "SendFLCam.vi"("madr"=w58, "data"=w59, "adadr"=w60) -> ()
            }
            frame #3 {
              w62 = u16 170  # data (hex)
              w63 = u8 4  # adadr (hex)
              # "Test pattern LSB regsiter A4 (TP7:TP0)\nAddress = 04h, Data = custom (8 bit)"
              n60 = global read "Globals.vi" "maddr of ADC"() -> (w61:u8)
              n61 = call "SendFLCam.vi"("madr"=w61, "data"=w62, "adadr"=w63) -> ()
            }
            frame #4 {
              # "register address pixel amount"
              # "pixel_für_aurora in cam_control_gerät"
              n62 = global read "Globals.vi" "PIXEL"() -> (w68:u32)
              n63 = global read "Globals.vi" "maddr of CAM"() -> (w65:u8)
              n64 = Multiply(x=w68, y=u32 1) -> (x*y=w67:u32)
              n65 = To Unsigned Word Integer(number=w67) -> (unsigned 16bit integer=w66:u16)
              n66 = call "SendFLCam.vi"("madr"=w65, "data"=w66, "adadr"=u8 1) -> ()
            }
          }
        }
        frame 3, Default {
          # "init routine for 3030"
          n67 = flat-sequence {
            frame #0 {
              n68 = global read "Globals.vi" "use DAC"() -> (w70:bool)
              n69 = case shown="True" w70 {
                frame False {
                }
                frame True {
                  w71 = u16 40960  # addr (hex)
                  w74 = fxp<+,4,4> 0.0  # feature (hex)
                  w75 = fxp<+,4,4> 0.0  # addr (hex)
                  w77 = fxp<+,4,4> 9.0  # ctrl (hex)
                  # "turn on internal reference voltage"
                  # "init DAC"
                  n70 = To Unsigned Byte Integer(number=w74) -> (unsigned 8bit integer=w73:u8)
                  n71 = To Unsigned Byte Integer(number=w75) -> (unsigned 8bit integer=w72:u8)
                  n72 = To Unsigned Byte Integer(number=w77) -> (unsigned 8bit integer=w76:u8)
                  n73 = call "SendFLCam_DAC.vi"("ctrl"=w76, "feature"=w73, "data"=w71, "addr"=w72) -> ()
                }
              }
            }
            frame #1 {
              # "set gain must be last in init sequence"
              n74 = global read "Globals.vi" "boards"() -> (w81:u32)
              n75 = call "SetAdGain_thread.vi"("gain"=u8 0, "board"=w81) -> ()  [unwired: 1 in]
              n76 = call "SetAdGain_thread.vi"("gain"=u8 0, "board"=u32 1) -> ()  [unwired: 1 in]
            }
          }
        }
      }
    }
    frame #2 {
      # "general init sequenz"
      n77 = flat-sequence {
        frame #0 {
          # "bit31 must be set for enabling DAT(add 0x80000000) to REG 0x20"
          # "is only valid for external trigger!"
          # "this examples shows how to set the DAT (delay after trigger)"
          n78 = Equal To 0?(x="DAT in 10ns") -> (x = 0?=w83:bool)
          n79 = case shown="True" w83 {
            tunnel: "DAT in 10ns" -> [w88 _]
            frame False {
              w85 = u32 32
              n80 = global read "Globals.vi" "boards"() -> (w87:u32)
              n81 = Add(x=u32 2147483648, y=w88) -> (x+y=w86:u32)
              n82 = call "WriteL_thread.vi"("val"=w86, "board"=w87, "offset"=w85) -> ()
              n83 = call "WriteL_thread.vi"("val"=w86, "board"=u32 1, "offset"=w85) -> ()
            }
            frame True {
              n84 = global read "Globals.vi" "boards"() -> (w94:u32)
              n85 = call "WriteL_thread.vi"("val"=u32 0, "board"=u32 1, "offset"=u32 32) -> ()
              n86 = call "WriteL_thread.vi"("val"=u32 0, "board"=w94, "offset"=u32 32) -> ()
            }
          }
        }
        frame #1 {
          w97 = FALSE
          w99 = 2
          n87 = global read "Globals.vi" "boards"() -> (w96:u32)
          n88 = case shown="1, Default" w96 {
            frame 2 {
              w102 = TRUE
              n89 = property on="Signalverlaufgraph" class="WFGraph (strict)"("Height"=u8 170) -> ()  [unwired: 2 in, 2 out]
              n90 = global write "Globals.vi" "board_sel"(u8 3) -> ()
              n91 = property on="boards recognised" class="DigNum (strict)"("Visible"=w102) -> ()  [unwired: 2 in, 2 out]
              n92 = property on="Board select\n1: board 1\n2: board 2\n3: both boards" class="DigNum (strict)"("Visible"=w102) -> ()  [unwired: 2 in, 2 out]
              n93 = property on="Signalverlaufgraph Board 2" class="WFGraph (strict)"("Visible"=w102) -> ()  [unwired: 2 in, 2 out]
            }
            frame 1, Default {
              w104 = FALSE
              n94 = global read "Globals.vi" "CAMCNT"() -> (w103:u32)
              n95 = case shown="2" w103 {
                frame 2 {
                  n96 = global write "Globals.vi" "board_sel"(u8 3) -> ()
                  n97 = property on="Signalverlaufgraph" class="WFGraph (strict)"("Height"=u8 170) -> ()  [unwired: 2 in, 2 out]
                  n98 = property on="Signalverlaufgraph Cam 2" class="WFGraph (strict)"("Visible"=TRUE) -> ()  [unwired: 2 in, 2 out]
                }
                frame 1, Default {
                  n99 = property on="Signalverlaufgraph" class="WFGraph (strict)"("Height"=400) -> ()  [unwired: 2 in, 2 out]
                  n100 = property on="Signalverlaufgraph Cam 2" class="WFGraph (strict)"("Visible"=FALSE) -> ()  [unwired: 2 in, 2 out]
                }
              }
              n101 = global write "Globals.vi" "board_sel"(u8 1) -> ()
              n102 = property on="Board select\n1: board 1\n2: board 2\n3: both boards" class="DigNum (strict)"("Visible"=w104) -> ()  [unwired: 2 in, 2 out]
              n103 = property on="Signalverlaufgraph Board 2" class="WFGraph (strict)"("Visible"=w104) -> ()  [unwired: 2 in, 2 out]
              n104 = property on="boards recognised" class="DigNum (strict)"("Visible"=w104) -> ()  [unwired: 2 in, 2 out]
            }
          }
          n105 = property on="sample" class="Slide (strict)"("DisabledEnum"=w99) -> ()  [unwired: 2 in, 2 out]
          n106 = property on="continuous" class="Bool (strict)"("DisabledEnum"=w99) -> ()  [unwired: 2 in, 2 out]
          n107 = property on="start" class="Bool (strict)"("DisabledEnum"=w99) -> ()  [unwired: 2 in, 2 out]
          n108 = property on="block" class="Slide (strict)"("DisabledEnum"=w99) -> ()  [unwired: 2 in, 2 out]
          n109 = property on="stop all" class="Bool (strict)"("DisabledEnum"=0) -> ()  [unwired: 2 in, 2 out]
          n110 = property on="continuous" class="Bool (strict)"("Value"=w97) -> ()  [unwired: 2 in, 2 out]
          n111 = property on="Measure ON" class="Bool (strict)"("Value"=w97) -> ()  [unwired: 2 in, 2 out]
        }
      }
    }
    frame #3 {
      # "display / hide chosen labview elements"
      n112 = global read "Globals.vi" "camera system select"() -> (w118:u8)
      n113 = global read "Globals.vi" "show ADC debug \ninterface"() -> (w116:bool)
      n114 = case shown="1, Default" w118 {
        tunnel: [FALSE FALSE TRUE] -> w114
        frame 1, Default {
        }
        frame 2 {
        }
        frame 3 {
        }
      }
      n115 = And(x=w114, y=w116) -> (x .and. y?=w117:bool)
      n116 = property on="ADC mode" class="RadioBtnsControl (strict)"("Visible"=w117) -> ()  [unwired: 2 in, 2 out]
      n117 = property on="custom pattern: 14bits (dec)" class="DigNum (strict)"("Visible"=w117) -> ()  [unwired: 2 in, 2 out]
      n118 = property on="custom pattern: 14bits (hex)" class="DigNum (strict)"("Visible"=w117) -> ()  [unwired: 2 in, 2 out]
      n119 = property on="data adr  0x25" class="DigNum (strict)"("Visible"=w117) -> ()  [unwired: 2 in, 2 out]
      n120 = property on="data adr  0x26" class="DigNum (strict)"("Visible"=w117) -> ()  [unwired: 2 in, 2 out]
      n121 = global read "Globals.vi" "use DAC"() -> (w115:bool)
      n122 = And(x=w114, y=w115) -> (x .and. y?=w113:bool)
      n123 = property on="Offset ADC 1" class="DigNum (strict)"("Visible"=w113) -> ()  [unwired: 2 in, 2 out]
      n124 = property on="Offset ADC 2" class="DigNum (strict)"("Visible"=w113) -> ()  [unwired: 2 in, 2 out]
      n125 = property on="Offset ADC 3" class="DigNum (strict)"("Visible"=w113) -> ()  [unwired: 2 in, 2 out]
      n126 = property on="Offset ADC 4" class="DigNum (strict)"("Visible"=w113) -> ()  [unwired: 2 in, 2 out]
      n127 = property on="Offset ADC 7" class="DigNum (strict)"("Visible"=w113) -> ()  [unwired: 2 in, 2 out]
      n128 = property on="Offset ADC 8" class="DigNum (strict)"("Visible"=w113) -> ()  [unwired: 2 in, 2 out]
      n129 = property on="Offset ADC 5" class="DigNum (strict)"("Visible"=w113) -> ()  [unwired: 2 in, 2 out]
      n130 = property on="Offset ADC 6" class="DigNum (strict)"("Visible"=w113) -> ()  [unwired: 2 in, 2 out]
      n131 = property on="send all" class="Bool (strict)"("Visible"=w113) -> ()  [unwired: 2 in, 2 out]
      n132 = global read "Globals.vi" "camera system select"() -> (w112:u8)
      n133 = case shown="1, Default" w112 {
        tunnel: [TRUE TRUE FALSE] -> w111
        frame 1, Default {
        }
        frame 2 {
        }
        frame 3 {
        }
      }
      n134 = property on="is FFT" class="Bool (strict)"("Visible"=w111) -> ()  [unwired: 2 in, 2 out]
      n135 = property on="IR gain" class="Bool (strict)"("Visible"=w111) -> ()  [unwired: 2 in, 2 out]
    }
    frame #4 {
      # "event structure while running"
      n136 = while {
        stop <- w126 stop-if-true
        n137 = event shown="[0] Timeout" {
          selector: _ -> [_ _ _ _ _ _ _ _ _ _ _ _ _ _ _ _ _ _ _ _]
          dyn-events: _ -> [_ _ _ _ _ _ _ _ _ _ _ _ _ _ _ _ _ _ _ _]
          timeout: 100 -> [_ _ _ _ _ _ _ _ _ _ _ _ _ _ _ _ _ _ _ _]
          tunnel: [_ _ _ _ _ _ _ _ w253 _ _ _ _ _ _ _ _ _ _ _] -> w126
          event Timeout {
            # "only refresh the frames if measure on"
            # "compares measure on signal from hardware with measure on lamp\nwhen diffrent than write new measure on value to lamp"
            # "timout excecutes every 100ms"
            # "userinfo of RAM, MeasureOB, Curr.Block and setting display event in cont mode"
            n138 = event-data() -> ()  [unwired: 1 in, 3 out]
            n139 = call "ReadB.vi"("Offset"=u32 64) -> ("Data"=w143:u8)
            n140 = call "FreeMemInfo.vi"() -> ("PhysicalSpace"=→"BUILT-IN\nRAM MB":dbl, "PhysicalFreeSpace"=→"FREE \nRAM MB":dbl)  [unwired: 1 in]
            n141 = Number To Boolean Array(number=w143) -> (Boolean array=w142:bool[])
            n142 = property on="Measure ON" class="Bool (strict)"() -> ("Value"=w137:bool)  [unwired: 2 in, 2 out]
            n143 = Index Array(array=w142, index=5) -> (element=w133:bool)
            n144 = Not Equal?(x=w137, y=w133) -> (x != y?=w136:bool)
            n145 = case shown="True" w136 {
              tunnel: w133 -> [_ w147]
              frame False {
              }
              frame True {
                n146 = property on="Measure ON" class="Bool (strict)"("Val(Sgnl)"=w147) -> ()  [unwired: 2 in, 2 out]
              }
            }
            n147 = property on="continuous" class="Bool (strict)"() -> ("DisabledEnum"=w130:T1)  [unwired: 2 in, 2 out]
            n148 = property on="continuous" class="Bool (strict)"() -> ("Value"=w139:bool)  [unwired: 2 in, 2 out]
            n149 = To Unsigned Byte Integer(number=w130) -> (unsigned 8bit integer=w131:u8)
            n150 = Equal?(x=w131, y=u8 0) -> (x = y?=w138:bool)
            n151 = And(x=w139, y=w138) -> (x .and. y?=w135:bool)
            n152 = And(x=w135, y=w133) -> (x .and. y?=w134:bool)
            n153 = call "ReadB.vi"("Offset"=u32 88) -> ("Data"=w128:u8)
            n154 = global read "Globals.vi" "CAMCNT"() -> (w127:u32)
            n155 = case shown="True" w134 {
              frame False {
              }
              frame True {
                # "refresh RMS.\nMaybe this is not a good style.\nIt's not clear to me which values are \nincluded to RMS measurement.\nBetter would be a refresh when all\nblocks are done."
                # "trigger the \ndisplay event"
                n156 = property on="rms_pixel" class="DigNum (strict)"() -> ("Value"=w148:u16)  [unwired: 2 in, 2 out]
                n157 = property on="sample" class="Slide (strict)"() -> ("Value"=w149:u32)  [unwired: 2 in, 2 out]
                n158 = property on="sample" class="Slide (strict)"("Val(Sgnl)"=w149) -> ()  [unwired: 2 in, 2 out]
                n159 = property on="rms_pixel" class="DigNum (strict)"("Val(Sgnl)"=w148) -> ()  [unwired: 2 in, 2 out]
              }
            }
            n160 = Divide(x=w128, y=w127) -> (x/y=→"curr.block":dbl)
          }
          event "Measure ON": Value Change {
            # "triggers on value change of measure on. this happens on start of measurement and after measurement\nwhen continuous: not after finishing all blocks, only when exiting measurement"
            n161 = event-data() -> ("NewVal"=w150:bool)  [unwired: 1 in, 5 out]
            n162 = property on="continuous" class="Bool (strict)"() -> ("Value"=w151:bool)  [unwired: 2 in, 2 out]
            n163 = And(x=w151, y=w150) -> (x .and. y?=w152:bool)
            n164 = case shown="False" w150 {
              frame False {
                n165 = property on="stop all" class="Bool (strict)"("DisabledEnum"=0) -> ()  [unwired: 2 in, 2 out]
              }
              frame True {
              }
            }
            n166 = case shown="True" w152 {
              frame False {
              }
              frame True {
                n167 = property on="stop all" class="Bool (strict)"("DisabledEnum"=2) -> ()  [unwired: 2 in, 2 out]
              }
            }
          }
          event "Board select\n1: board 1\n2: board 2\n3: both boards": Value Change {
            # "selecting number of cams"
            n168 = event-data() -> ()  [unwired: 1 in, 6 out]
            n169 = global read "Globals.vi" "boards"() -> (w155:u32)
            n170 = case shown="2" w155 {
              frame 0, Default {
              }
              frame 2 {
                n171 = global write "Globals.vi" "board_sel"("Board select\n1: board 1\n2: board 2\n3: both boards") -> ()
              }
            }
          }
          event "continuous": Value Change {
            # "setting continuos mode"
            n172 = event-data() -> ()  [unwired: 1 in, 6 out]
            n173 = case shown="True" "continuous" {
              tunnel: [u8 0 u8 1] -> w157
              frame False {
              }
              frame True {
              }
            }
            n174 = call "contFFLoop.vi"("Numeric"=w157) -> ()  [unwired: 1 in]
          }
          event "alloc mem": Value Change {
            w165 = 0
            # "update params"
            # "Setup DMA"
            n175 = event-data() -> ()  [unwired: 1 in, 6 out]
            n176 = global read "Globals.vi" "CAMCNT"() -> (w164:u32)
            n177 = global read "Globals.vi" "nob"() -> (w162:u32)
            n178 = global read "Globals.vi" "nos"() -> (w163:u32)
            n179 = To Unsigned Long Integer(number=w164) -> (unsigned 32bit integer=w161:u32)
            n180 = global read "Globals.vi" "boards"() -> (w168:u32)
            n181 = case shown="2" w168 {
              selector: w168 -> [_ w170]
              tunnel: w163 -> [_ w171]
              tunnel: w162 -> [_ w172]
              tunnel: w161 -> [_ w169]
              frame 1, Default {
              }
              frame 2 {
                # "Setup DMA"
                n182 = call "SetupDMA_thread.vi"("camcnt"=w169, "blocks"=w172, "nos"=w171, "Drv"=w170) -> ()  [unwired: 1 in]
              }
            }
            n183 = call "SetupDMA_thread.vi"("camcnt"=w161, "blocks"=w162, "nos"=w163, "Drv"=u32 1) -> ()  [unwired: 1 in]
            n184 = property on="exposuretime[ms]" class="DigNum (strict)"() -> ("Value"=w167:dbl)  [unwired: 2 in, 2 out]
            n185 = property on="exposuretime[ms]" class="DigNum (strict)"("Val(Sgnl)"=w167) -> ()  [unwired: 2 in, 2 out]
            n186 = property on="continuous" class="Bool (strict)"("DisabledEnum"=w165) -> ()  [unwired: 2 in, 2 out]
            n187 = property on="block" class="Slide (strict)"("DisabledEnum"=w165) -> ()  [unwired: 2 in, 2 out]
            n188 = property on="sample" class="Slide (strict)"("DisabledEnum"=w165) -> ()  [unwired: 2 in, 2 out]
            n189 = property on="start" class="Bool (strict)"("DisabledEnum"=w165) -> ()  [unwired: 2 in, 2 out]
          }
          event "start": Mouse Down {
            # "start measurement"
            # "only 1st PCI board is used for ext. trig."
            # "ext. block trig\n0: internal: Space\n1: PCI \"I\"\n2: S1\n3: S2"
            # "block trigger 0/1\n0: internal -> next block is started immediately \n1: external -> each block has an own trigger"
            n190 = event-data() -> ()  [unwired: 1 in, 8 out]
            n191 = global read "Globals.vi" "exp time"() -> (w179:dbl)
            n192 = Multiply(x=1000.0, y=w179) -> (x*y=w181:dbl)
            n193 = global read "Globals.vi" "board_sel"() -> (w175:u8)
            n194 = To Unsigned Long Integer(number=w181) -> (unsigned 32bit integer=w177:u32)
            n195 = case shown="True" "extTrig" {
              tunnel: [u8 0 u8 1] -> w174
              frame False {
              }
              frame True {
              }
            }
            n196 = call "ReadFFLoop_thread.vi"("blocktrigger"=u8 0, "btrig_ch"=u8 0, "ExtTrig"=w174, "cam_sel"=w175, "exptus"=w177) -> ()  [unwired: 1 in]
          }
          event "sample", "block": Value Change {
            w200 = u32 1
            # "when selecting a value\nbigger than possible\nnos or nob, a dummy \nvalue \"1\" is chosen\n\nTODO:\ninsert error handling\nwith lower values than 1"
            # "display"
            n197 = event-data() -> ()  [unwired: 1 in, 6 out]
            n198 = global read "Globals.vi" "boards"() -> (w201:u32)
            n199 = global read "Globals.vi" "nob"() -> (w192:u32)
            n200 = global read "Globals.vi" "nos"() -> (w199:u32)
            n201 = Greater Or Equal?(x=w192, y="block") -> (x >= y?=w195:bool)
            n202 = Greater Or Equal?(x=w199, y="sample") -> (x >= y?=w198:bool)
            n203 = case shown="True" w195 {
              tunnel: [u32 1 w216] -> w194
              tunnel: "block" -> [_ w216]
              frame False {
                n204 = call "Display Message to User"() -> ()  [unwired: 10 in, 2 out]
              }
              frame True {
              }
            }
            n205 = case shown="False" w198 {
              tunnel: [u32 1 w218] -> w197
              tunnel: "sample" -> [_ w218]
              frame False {
                n206 = call "Display Message to User2"() -> ()  [unwired: 10 in, 2 out]
              }
              frame True {
              }
            }
            n207 = global read "Globals.vi" "CAMCNT"() -> (w185:u32)
            n208 = global read "Globals.vi" "PIXEL"() -> (w189:u32)
            n209 = Subtract(x=w197, y=w200) -> (x-y=w186:u32)
            n210 = Subtract(x=w194, y=w200) -> (x-y=w187:u32)
            n211 = case shown="2" w201 {
              selector: w201 -> [_ w223]
              tunnel: w186 -> [_ w224]
              tunnel: w187 -> [_ w221]
              frame 0, Default {
              }
              frame 2 {
                n212 = global read "Globals.vi" "PIXEL"() -> (w219:u32)
                n213 = To Long Integer(number=w219) -> (32bit integer=w220:i32)
                n214 = Initialize Array(u16 100, w220) -> (w226:u16[])
                n215 = call "ReturnFrame.vi"("Data Values In"=w226, "curr_nob"=w221, "curr_nos"=w224, "Drv"=w223) -> ("Data Values Out"=→"Signalverlaufgraph Board 2":u16[])  [unwired: 1 in]
              }
            }
            n216 = To Long Integer(number=w189) -> (32bit integer=w190:i32)
            n217 = Initialize Array(u16 100, w190) -> (w204:u16[])
            n218 = Multiply(x=w185, y=w186) -> (x*y=w184:u32)
            n219 = call "ReturnFrame.vi"("Data Values In"=w204, "curr_nob"=w187, "curr_nos"=w184, "Drv"=u32 1) -> ("Data Values Out"=→"Signalverlaufgraph":u16[])  [unwired: 1 in]
            n220 = global read "Globals.vi" "CAMCNT"() -> (w188:u32)
            n221 = case shown="2" w188 {
              tunnel: w187 -> [_ w208]
              tunnel: w184 -> [_ w206]
              frame 1, Default {
              }
              frame 2 {
                n222 = Add(x=w206, y=u32 1) -> (x+y=w207:u32)
                n223 = global read "Globals.vi" "PIXEL"() -> (w213:u32)
                n224 = To Long Integer(number=w213) -> (32bit integer=w212:i32)
                n225 = Initialize Array(u16 100, w212) -> (w209:u16[])
                n226 = call "ReturnFrame.vi"("Data Values In"=w209, "curr_nob"=w208, "curr_nos"=w207, "Drv"=u32 1) -> ("Data Values Out"=→"Signalverlaufgraph Cam 2":u16[])  [unwired: 1 in]
              }
            }
          }
          event "no.of samples (nos)", "no.of blocks (nob)\npress enter", "exposuretime[ms]": Value Change {
            # "calculation of MB RAM an SEC and setting scale max"
            # "MB"
            # "ushort"
            n227 = event-data() -> ()  [unwired: 1 in, 7 out]
            n228 = global read "Globals.vi" "PIXEL"() -> (w252:u32)
            n229 = Multiply(x="no.of samples (nos)", y=w252) -> (x*y=w250:u32)
            n230 = Multiply(x=w250, y=u32 2) -> (x*y=w230:u32)
            n231 = global read "Globals.vi" "boards"() -> (w251:u32)
            n232 = global read "Globals.vi" "CAMCNT"() -> (w229:u32)
            n233 = global read "Globals.vi" "nos"() -> (w234:u32)
            n234 = global read "Globals.vi" "nob"() -> (w232:u32)
            n235 = To Unsigned Long Integer(number=w229) -> (unsigned 32bit integer=w228:u32)
            n236 = Multiply(x=w228, y=w230) -> (x*y=w227:u32)
            n237 = Multiply(x=w227, y=w251) -> (x*y=w240:u32)
            n238 = To Double Precision Float(number=w240) -> (double precision float=w239:dbl)
            n239 = To Double Precision Float(number=w234) -> (double precision float=w233:dbl)
            n240 = Divide(x=w239, y=1048576.0) -> (x/y=w242:dbl)
            n241 = To Double Precision Float(number=w232) -> (double precision float=w231:dbl)
            n242 = To Double Precision Float(number="no.of blocks (nob)\npress enter") -> (double precision float=w237:dbl)
            n243 = property on="sample" class="Slide (strict)"("Scale.Maximum"=w233) -> ()  [unwired: 2 in, 2 out]
            n244 = property on="block" class="Slide (strict)"("Scale.Maximum"=w231) -> ()  [unwired: 2 in, 2 out]
            n245 = Multiply(x=w242, y=w237) -> (x*y=→"MB RAM":dbl)
            n246 = global write "Globals.vi" "nos"("no.of samples (nos)") -> ()
            n247 = Multiply(x="no.of samples (nos)", y="no.of blocks (nob)\npress enter") -> (x*y=w235:u32)
            n248 = global write "Globals.vi" "nob"("no.of blocks (nob)\npress enter") -> ()
            n249 = To Double Precision Float(number=w235) -> (double precision float=w236:dbl)
            n250 = global write "Globals.vi" "exp time"("exposuretime[ms]") -> ()
            n251 = Multiply(x="exposuretime[ms]", y=w236) -> (x*y=w248:dbl)
            n252 = Divide(x=w248, y=1000.0) -> (x/y=→"SEC":dbl)
          }
          event "stop all": Value Change {
            # "exit"
            n253 = event-data() -> ()  [unwired: 1 in, 6 out]
            n254 = stacked-sequence {
              tunnel: [_ TRUE] -> w253
              frame #0 {
                n255 = call "FFStop.vi"() -> ()  [unwired: 1 in]
              }
              frame #1 {
                # "do not omit, or next call of driver will go wrong."
                n256 = call "Exit.vi"() -> ()  [unwired: 1 in]
              }
            }
          }
          event "rms_pixel": Value Change {
            # "one array with all values (except first 10)\nat index Pixel from all blocks"
            n257 = event-data() -> ()  [unwired: 1 in, 6 out]
            n258 = global read "Globals.vi" "nos"() -> (w259:u32)
            n259 = global read "Globals.vi" "nob"() -> (w260:u32)
            n260 = for {
              N: w260 -> [_]
              tunnel: w259 -> [w261]
              tunnel: [w263] -> w256 mode=concatenating
              i -> [w267]
              # "delete first 10 values"
              # "array of all values\nat index Pixel"
              n261 = To Long Integer(number=w261) -> (32bit integer=w262:i32)
              n262 = for {
                N: w262 -> [_]
                tunnel: w267 -> [w272]
                tunnel: [w276] -> w264 mode=indexing
                i -> [w274]
                # "use only value at index \"Pixel\""
                # "init array of size PIXEL\nwith value 100"
                n263 = global read "Globals.vi" "PIXEL"() -> (w268:u32)
                n264 = To Long Integer(number=w268) -> (32bit integer=w269:i32)
                n265 = To Unsigned Long Integer(number=w272) -> (unsigned 32bit integer=w273:u32)
                n266 = To Unsigned Long Integer(number=w274) -> (unsigned 32bit integer=w275:u32)
                n267 = Initialize Array(u16 100, w269) -> (w278:u16[])
                n268 = call "ReturnFrame.vi"("Data Values In"=w278, "curr_nob"=w273, "curr_nos"=w275, "Drv"=u32 1) -> ("Data Values Out"=w277:u16[])  [unwired: 1 in]
                n269 = To Long Integer(number="rms_pixel") -> (32bit integer=w270:i32)
                n270 = Index Array(array=w277, index=w270) -> (element=w276:u16)
              }
              n271 = Delete From Array(array=w264, length=10, index=0) -> (array with subset deleted=w263:u16[])  [unwired: 1 out]
            }
            n272 = To Double Precision Float(number=w256) -> (double precision float=w255:dbl[])
            n273 = call <vilib>:"Std Deviation and Variance.vi"("X"=w255) -> ("mean"=→"mean":dbl, "standard deviation"=→"tRMS":dbl)  [unwired: 1 in, 1 out]
          }
          event "ADC mode", "custom pattern: 14bits (hex)": Value Change {
            n274 = event-data() -> ()  [unwired: 1 in, 6 out]
            n275 = case shown="\"1\"" "ADC mode" {
              frame "1" {
                w305 = u8 38  # adadr (hex)
                w306 = u8 37  # adadr (hex)
                # "Custom Pattern"
                n276 = Number To Boolean Array(number="custom pattern: 14bits (hex)") -> (Boolean array=w304:bool[])
                n277 = Number To Boolean Array(number="custom pattern: 14bits (hex)") -> (Boolean array=w301:bool[])
                n278 = Number To Boolean Array(number=fxp<+,12,12> 4.0) -> (Boolean array=w296:bool[])
                n279 = Array Subset(array=w304, index=0, length=12) -> (w286:bool[])
                n280 = Array Subset(array=w301, index=12, length=2) -> (w297:bool[])
                n281 = Insert Into Array(array=w296, index=0, new element=w297) -> (w294:bool[])
                n282 = Number To Boolean Array(number=fxp<+,4,4> 0.0) -> (Boolean array=w287:bool[])
                n283 = Boolean Array To Number(Boolean array=w294) -> (number=w293:u32)
                n284 = Insert Into Array(array=w286, index=0, new element=w287) -> (w285:bool[])
                n285 = To Unsigned Word Integer(number=w293) -> (unsigned 16bit integer=w289:u16)
                "data adr  0x25" <- w289
                n286 = Boolean Array To Number(Boolean array=w285) -> (number=w290:u32)
                n287 = To Unsigned Word Integer(number=w290) -> (unsigned 16bit integer=w288:u16)
                "data adr  0x26" <- w288
                n288 = global read "Globals.vi" "maddr of ADC"() -> (w282:u8)
                n289 = global read "Globals.vi" "maddr of ADC"() -> (w283:u8)
                n290 = call "SendFLCam.vi"("madr"=w283, "data"=w289, "adadr"=w306) -> ()
                n291 = call "SendFLCam.vi"("madr"=w282, "data"=w288, "adadr"=w305) -> ()
                "custom pattern: 14bits (dec)" <- "custom pattern: 14bits (hex)"
              }
              frame "2" {
                w308 = u16 0  # data (hex)
                w309 = u16 64  # data (hex)
                w310 = u8 37  # adadr (hex)
                # "Ramp"
                n292 = global read "Globals.vi" "maddr of ADC"() -> (w307:u8)
                n293 = call "SendFLCam.vi"("madr"=w307, "data"=w309, "adadr"=w310) -> ()
                n294 = property on="data adr  0x26" class="DigNum (strict)"("Val(Sgnl)"=w308) -> ()  [unwired: 2 in, 2 out]
                n295 = property on="data adr  0x25" class="DigNum (strict)"("Val(Sgnl)"=w309) -> ()  [unwired: 2 in, 2 out]
              }
              frame "3" {
                w316 = u16 1  # data
                w317 = u8 0  # adadr (hex)
                w315 = u16 0  # data
                w318 = u8 38  # adadr (hex)
                w314 = u16 0  # data
                w319 = u8 37  # adadr (hex)
                # "Normal Mode"
                n296 = global read "Globals.vi" "maddr of ADC"() -> (w312:u8)
                n297 = global read "Globals.vi" "maddr of ADC"() -> (w313:u8)
                n298 = global read "Globals.vi" "maddr of ADC"() -> (w311:u8)
                n299 = call "SendFLCam.vi"("madr"=w312, "data"=w315, "adadr"=w318) -> ()
                n300 = call "SendFLCam.vi"("madr"=w313, "data"=w316, "adadr"=w317) -> ()
                n301 = call "SendFLCam.vi"("madr"=w311, "data"=w314, "adadr"=w319) -> ()
                n302 = property on="data adr  0x26" class="DigNum (strict)"("Val(Sgnl)"=w315) -> ()  [unwired: 2 in, 2 out]
                n303 = property on="data adr  0x25" class="DigNum (strict)"("Val(Sgnl)"=w314) -> ()  [unwired: 2 in, 2 out]
              }
            }
          }
          event "Offset ADC 4": Value Change {
            w324 = fxp<+,4,4> 0.0  # feature (hex)
            w323 = fxp<+,4,4> 0.0  # addr (hex)
            w321 = fxp<+,4,4> 3.0  # ctrl (hex)
            # "Register CHA"
            # "ctrl: write and update DAC register"
            n304 = event-data() -> ()  [unwired: 1 in, 6 out]
            n305 = To Unsigned Byte Integer(number=w324) -> (unsigned 8bit integer=w325:u8)
            n306 = To Unsigned Byte Integer(number=w323) -> (unsigned 8bit integer=w326:u8)
            n307 = To Unsigned Byte Integer(number=w321) -> (unsigned 8bit integer=w322:u8)
            n308 = call "SendFLCam_DAC.vi"("ctrl"=w322, "feature"=w325, "data"="Offset ADC 4", "addr"=w326) -> ()
          }
          event "Offset ADC 5": Value Change {
            w330 = fxp<+,4,4> 0.0  # feature (hex)
            w329 = fxp<+,4,4> 1.0  # addr (hex)
            w327 = fxp<+,4,4> 3.0  # ctrl (hex)
            # "Register CHB"
            # "ctrl: write and update DAC register"
            n309 = event-data() -> ()  [unwired: 1 in, 6 out]
            n310 = To Unsigned Byte Integer(number=w330) -> (unsigned 8bit integer=w331:u8)
            n311 = To Unsigned Byte Integer(number=w329) -> (unsigned 8bit integer=w332:u8)
            n312 = To Unsigned Byte Integer(number=w327) -> (unsigned 8bit integer=w328:u8)
            n313 = call "SendFLCam_DAC.vi"("ctrl"=w328, "feature"=w331, "data"="Offset ADC 5", "addr"=w332) -> ()
          }
          event "Offset ADC 1": Value Change {
            w337 = fxp<+,4,4> 0.0  # feature (hex)
            w336 = fxp<+,4,4> 2.0  # addr (hex)
            w334 = fxp<+,4,4> 3.0  # ctrl (hex)
            # "Register CHC"
            # "ctrl: write and update DAC register"
            n314 = event-data() -> ()  [unwired: 1 in, 6 out]
            n315 = To Unsigned Byte Integer(number=w337) -> (unsigned 8bit integer=w338:u8)
            n316 = To Unsigned Byte Integer(number=w336) -> (unsigned 8bit integer=w339:u8)
            n317 = To Unsigned Byte Integer(number=w334) -> (unsigned 8bit integer=w335:u8)
            n318 = call "SendFLCam_DAC.vi"("ctrl"=w335, "feature"=w338, "data"="Offset ADC 1", "addr"=w339) -> ()
          }
          event "Offset ADC 6": Value Change {
            w344 = fxp<+,4,4> 0.0  # feature (hex)
            w343 = fxp<+,4,4> 3.0  # addr (hex)
            w341 = fxp<+,4,4> 3.0  # ctrl (hex)
            # "Register CHD"
            # "ctrl: write and update DAC register"
            n319 = event-data() -> ()  [unwired: 1 in, 6 out]
            n320 = To Unsigned Byte Integer(number=w344) -> (unsigned 8bit integer=w345:u8)
            n321 = To Unsigned Byte Integer(number=w343) -> (unsigned 8bit integer=w346:u8)
            n322 = To Unsigned Byte Integer(number=w341) -> (unsigned 8bit integer=w342:u8)
            n323 = call "SendFLCam_DAC.vi"("ctrl"=w342, "feature"=w345, "data"="Offset ADC 6", "addr"=w346) -> ()
          }
          event "Offset ADC 2": Value Change {
            w351 = fxp<+,4,4> 0.0  # feature (hex)
            w350 = fxp<+,4,4> 4.0  # addr (hex)
            w348 = fxp<+,4,4> 3.0  # ctrl (hex)
            # "Register CHE"
            # "ctrl: write and update DAC register"
            n324 = event-data() -> ()  [unwired: 1 in, 6 out]
            n325 = To Unsigned Byte Integer(number=w351) -> (unsigned 8bit integer=w352:u8)
            n326 = To Unsigned Byte Integer(number=w350) -> (unsigned 8bit integer=w353:u8)
            n327 = To Unsigned Byte Integer(number=w348) -> (unsigned 8bit integer=w349:u8)
            n328 = call "SendFLCam_DAC.vi"("ctrl"=w349, "feature"=w352, "data"="Offset ADC 2", "addr"=w353) -> ()
          }
          event "Offset ADC 7": Value Change {
            w358 = fxp<+,4,4> 0.0  # feature (hex)
            w357 = fxp<+,4,4> 5.0  # addr (hex)
            w355 = fxp<+,4,4> 3.0  # ctrl (hex)
            # "Register CHF"
            # "ctrl: write and update DAC register"
            n329 = event-data() -> ()  [unwired: 1 in, 6 out]
            n330 = To Unsigned Byte Integer(number=w358) -> (unsigned 8bit integer=w359:u8)
            n331 = To Unsigned Byte Integer(number=w357) -> (unsigned 8bit integer=w360:u8)
            n332 = To Unsigned Byte Integer(number=w355) -> (unsigned 8bit integer=w356:u8)
            n333 = call "SendFLCam_DAC.vi"("ctrl"=w356, "feature"=w359, "data"="Offset ADC 7", "addr"=w360) -> ()
          }
          event "Offset ADC 3": Value Change {
            w365 = fxp<+,4,4> 0.0  # feature (hex)
            w364 = fxp<+,4,4> 6.0  # addr (hex)
            w362 = fxp<+,4,4> 3.0  # ctrl (hex)
            # "Register CHG"
            # "ctrl: write and update DAC register"
            n334 = event-data() -> ()  [unwired: 1 in, 6 out]
            n335 = To Unsigned Byte Integer(number=w365) -> (unsigned 8bit integer=w366:u8)
            n336 = To Unsigned Byte Integer(number=w364) -> (unsigned 8bit integer=w367:u8)
            n337 = To Unsigned Byte Integer(number=w362) -> (unsigned 8bit integer=w363:u8)
            n338 = call "SendFLCam_DAC.vi"("ctrl"=w363, "feature"=w366, "data"="Offset ADC 3", "addr"=w367) -> ()
          }
          event "Offset ADC 8": Value Change {
            w372 = fxp<+,4,4> 0.0  # feature (hex)
            w371 = fxp<+,4,4> 7.0  # addr (hex)
            w369 = fxp<+,4,4> 3.0  # ctrl (hex)
            # "Register CHH"
            # "ctrl: write and update DAC register"
            n339 = event-data() -> ()  [unwired: 1 in, 6 out]
            n340 = To Unsigned Byte Integer(number=w372) -> (unsigned 8bit integer=w373:u8)
            n341 = To Unsigned Byte Integer(number=w371) -> (unsigned 8bit integer=w374:u8)
            n342 = To Unsigned Byte Integer(number=w369) -> (unsigned 8bit integer=w370:u8)
            n343 = call "SendFLCam_DAC.vi"("ctrl"=w370, "feature"=w373, "data"="Offset ADC 8", "addr"=w374) -> ()
          }
          event "send all": Value Change {
            n344 = event-data() -> ()  [unwired: 1 in, 6 out]
            n345 = property on="Offset ADC 1" class="DigNum (strict)"() -> ("Value"=w376:u16)  [unwired: 2 in, 2 out]
            n346 = property on="Offset ADC 4" class="DigNum (strict)"() -> ("Value"=w379:u16)  [unwired: 2 in, 2 out]
            n347 = property on="Offset ADC 2" class="DigNum (strict)"() -> ("Value"=w377:u16)  [unwired: 2 in, 2 out]
            n348 = property on="Offset ADC 3" class="DigNum (strict)"() -> ("Value"=w378:u16)  [unwired: 2 in, 2 out]
            n349 = property on="Offset ADC 1" class="DigNum (strict)"("Val(Sgnl)"=w376) -> ()  [unwired: 2 in, 2 out]
            n350 = property on="Offset ADC 4" class="DigNum (strict)"("Val(Sgnl)"=w379) -> ()  [unwired: 2 in, 2 out]
            n351 = property on="Offset ADC 2" class="DigNum (strict)"("Val(Sgnl)"=w377) -> ()  [unwired: 2 in, 2 out]
            n352 = property on="Offset ADC 3" class="DigNum (strict)"("Val(Sgnl)"=w378) -> ()  [unwired: 2 in, 2 out]
            n353 = property on="Offset ADC 8" class="DigNum (strict)"() -> ("Value"=w383:u16)  [unwired: 2 in, 2 out]
            n354 = property on="Offset ADC 5" class="DigNum (strict)"() -> ("Value"=w380:u16)  [unwired: 2 in, 2 out]
            n355 = property on="Offset ADC 7" class="DigNum (strict)"() -> ("Value"=w382:u16)  [unwired: 2 in, 2 out]
            n356 = property on="Offset ADC 6" class="DigNum (strict)"() -> ("Value"=w381:u16)  [unwired: 2 in, 2 out]
            n357 = property on="Offset ADC 8" class="DigNum (strict)"("Val(Sgnl)"=w383) -> ()  [unwired: 2 in, 2 out]
            n358 = property on="Offset ADC 5" class="DigNum (strict)"("Val(Sgnl)"=w380) -> ()  [unwired: 2 in, 2 out]
            n359 = property on="Offset ADC 7" class="DigNum (strict)"("Val(Sgnl)"=w382) -> ()  [unwired: 2 in, 2 out]
            n360 = property on="Offset ADC 6" class="DigNum (strict)"("Val(Sgnl)"=w381) -> ()  [unwired: 2 in, 2 out]
          }
        }
      }
    }
  }
  n361 = property on="sample" class="Slide (strict)"("DisabledEnum"=w1) -> ()  [unwired: 2 in, 2 out]
  n362 = property on="start" class="Bool (strict)"("DisabledEnum"=w1) -> ()  [unwired: 2 in, 2 out]
  n363 = property on="block" class="Slide (strict)"("DisabledEnum"=w1) -> ()  [unwired: 2 in, 2 out]
